vi "Two Parameter Marco Reparam EB only.vi"() -> ()   [LabVIEW 2015]
uses:
  <vilib>/Platform/TimedLoop/XDataNode/timing_clust.ctl
  <vilib>/Platform/TimedLoop/XDataNode/nitl_modes.ctl
  <vilib>/Platform/TimedLoop/XDataNode/wakeup.ctl
  <vilib>/DAQmx/read.llb/DAQmx Read (Analog DBL 1Chan 1Samp).vi
  <vilib>/DAQmx/read.llb/DAQmx Read (Analog 1D DBL NChan 1Samp).vi
  <vilib>/DAQmx/create/channels.llb/DAQmx Create Channel (AI-Voltage-Basic).vi
  <vilib>/Enthought/Python Integration Toolkit/api/Unpack Double.vi
  <vilib>/DAQmx/miscellaneous.llb/DAQmx Fill In Error Info.vi
  <vilib>/Platform/TimedLoop/XDataNode/XDataNode.xnode
  Program Files/neMESYS_SDK/neMESYS LabVIEW Kit/neMESYS LabVIEW Integration Kit.lvlib
  <vilib>/Platform/TimedLoop/XDataNode/XDNodeRunTimeDep.lvlib
  Conor/Temp CN7500/Omega CN7500/Omega CN7500.lvlib
  <vilib>/Enthought/Python Integration Toolkit/Python Integration Toolkit.lvlib
panel:
  out "Exp 10":bool
  out "Temp 3":dbl
  out "Flow 3":dbl
  out "Conc 3":dbl
  out "C BAcid 2":dbl
  out "C EB 2":dbl
  in  "Temp 3":dbl
  in  "Conc 3":dbl
  in  "Flow 3":dbl
  in  "LogFileName must end with .txt":string
  out "Param 1 8":dbl
  out "T value 1 8":dbl
  out "Param 2 8":dbl
  out "T value 2 8":dbl
  out "T Ref 8":dbl
  out "Correlation 8":dbl
  out "X2 8":dbl
  out "X2 ref 8":dbl
  out "Temp 9":dbl
  out "Flow 9":dbl
  out "Conc 9":dbl
  out "C BAcid 8":dbl
  out "C EB 8":dbl
  out "Exp 9":bool
  out "Param 1 7":dbl
  out "T value 1 7":dbl
  out "Param 2 7":dbl
  out "T value 2 7":dbl
  out "T Ref 7":dbl
  out "Correlation 7":dbl
  out "X2 7":dbl
  out "X2 ref 7":dbl
  out "Temp 8":dbl
  out "Flow 8":dbl
  out "Conc 8":dbl
  out "C BAcid 7":dbl
  out "C EB 7":dbl
  out "Exp 8":bool
  out "Param 1 6":dbl
  out "T value 1 6":dbl
  out "Param 2 6":dbl
  out "T value 2 6":dbl
  out "T Ref 6":dbl
  out "Correlation 6":dbl
  out "X2 6":dbl
  out "X2 ref 6":dbl
  out "Temp 7":dbl
  out "Flow 7":dbl
  out "Conc 7":dbl
  out "C BAcid 6":dbl
  out "C EB 6":dbl
  out "Exp 7":bool
  out "Param 1 5":dbl
  out "T value 1 5":dbl
  out "Param 2 5":dbl
  out "T value 2 5":dbl
  out "T Ref 5":dbl
  out "Correlation 5":dbl
  out "X2 5":dbl
  out "X2 ref 5":dbl
  out "Temp 6":dbl
  out "Flow 6":dbl
  out "Conc 6":dbl
  out "C BAcid 5":dbl
  out "C EB 5":dbl
  out "Exp 6":bool
  out "Param 1 4":dbl
  out "T value 1 4":dbl
  out "Param 2 4":dbl
  out "T value 2 4":dbl
  out "T Ref 4":dbl
  out "Correlation 4":dbl
  out "X2 4":dbl
  out "X2 ref 4":dbl
  out "Temp 5":dbl
  out "Flow 5":dbl
  out "Conc 5":dbl
  out "C BAcid 4":dbl
  out "C EB 4":dbl
  out "Exp 5":bool
  out "Param 1 3":dbl
  out "T value 1 3":dbl
  out "Param 2 3":dbl
  out "T value 2 3":dbl
  out "T Ref 3":dbl
  out "Correlation 3":dbl
  out "X2 3":dbl
  out "X2 ref 3":dbl
  out "Temp 4":dbl
  out "Flow 4":dbl
  out "Conc 4":dbl
  out "C BAcid 3":dbl
  out "C EB 3":dbl
  out "Exp 4":bool
  out "Conc 10":dbl
  out "Flow 10":dbl
  out "Temp 10":dbl
  in  "Design Criteria A or D or E or SV":string
  in  "Reparameterise? ON or OFF":string
  out "Exp 2":bool
  out "C EB 1":dbl
  out "C BAcid 1":dbl
  out "X2 ref 9":dbl
  out "X2 9":dbl
  out "Exp 2":bool
  out "Liquid Inlet Pressure (bar g)":dbl
  in  "Liquid P sensor Terminal Configuration":i32(ring)=-1 items=["default"=-1, "RSE"=10083, "NRSE"=10078, "Differential"=10106, "Pseudodifferential"=12529]
  in  "Liquid P sensor Physical Channel":tag="Dev1/ai0"
  in  "Temp 2":dbl
  in  "Conc 2":dbl
  in  "Flow 2":dbl
  out "Correlation 9":dbl
  out "T Ref 9":dbl
  out "Exp Finish":bool
  out "Exp 1":bool
  out "Exp 0":bool
  out "Conc 1":dbl
  out "Flow 1":dbl
  out "Temp 1":dbl
  out "Conc 2":dbl
  out "Flow 2":dbl
  out "Temp 2":dbl
  out "Param 1 9":dbl
  out "T value 1 9":dbl
  out "Param 2 9":dbl
  out "T value 2 9":dbl
  out "C BAcid 9":dbl
  out "C EB 9":dbl
  in  "Result file name must end with .xlsx":string
  in  "HPLC file Name, dont need extension":string
  out "Desired Conc Not Possible":bool
  in  "Safety or Emergency Syringe Control":bool
  out "Feed Concentration (M)":dbl
  out "Total Flowrate (uL/min)":dbl
  out "Gas Back Pressure (barg)":dbl
  in  "Shut down in empty?\nLeft off, right on":bool
  in  "Clear":bool
  out "Safety Shut Down Pressure (barg)":dbl
  out "Calculated Pressure":dbl[](graph)
  out "Safety Shut Down Temp":dbl
  out "Actual Temp (oC)":dbl
  out "Temperature":dynamicdata(graph)
  out "Temp Set Point (oC)":dbl
  in  "Temp 1":dbl
  in  "Temp 0":dbl
  in  "Update Temperature Set Point":bool
  in  "Automated Experiments or Direct Control":bool
  in  "Set Point (oC)":dbl
  out "loop ind":dbl
  in  "Stop everything":bool
  in  "Skip Exp":bool
  in  "Minutes between Exp":dbl min=0.0 step=0.05
  in  "Refill 4":bool
  in  "Refill 3":bool
  in  "Refill 2":bool
  in  "Refill 1":bool
  in  "Empty 4":bool
  in  "Empty 3":bool
  in  "Empty 2":bool
  in  "Empty 1":bool
  in  "Calibrate 4":bool
  in  "Calibrate 3":bool
  in  "Calibrate 2":bool
  in  "Calibrate 1":bool
  in  "Stop Dose 4":bool
  in  "Stop Dose 3":bool
  in  "Stop Dose 2":bool
  in  "Stop Dose 1":bool
  in  "Flow 1":dbl
  in  "Conc 1":dbl
  in  "Flow 0":dbl
  in  "Conc 0":dbl
  in  "Generate Flow":bool
  in  "Set Flowrate 1":dbl
  in  "Set Flowrate 2":dbl
  in  "Set Flowrate 3":dbl
  in  "Set Flowrate 4":dbl
  in  "High Conc":dbl min=0.0 max=2.0
  in  "Low Conc":dbl min=0.0 max=2.0
  out "Volumetric Fraction Acid":dbl min=0.0 max=1.0
  out "Syringe Level 4":dbl(slide) scale=0.0..5500.0
  out "Syringe Level 3":dbl(slide) scale=0.0..5500.0
  out "Syringe Level 2":dbl(slide) scale=0.0..5500.0
  out "Syringe Level 1":dbl(slide) scale=0.0..5500.0
  out "Flowrate 4 Ethanol":dbl
  out "Flowrate 3 Acid":dbl
  out "Flowrate 2 High":dbl
  out "Flowrate 1 Low":dbl
  # "Pre Planned Experiments"
  # "Conducted Experiments Set Points"
  # "Safety (start and end)"
  # "Current Conditions"
  # "(uL/min)"
  # "Coerced to nearest possible"
  # "Experimental Info"
  # "Acid must be between 0 and 1, normally 0.1 for 10%"
  # "Direct Control"
  # "Unit of Gas Flow NmL/min"
  # "I swapped syringe 1 and 2, so now 2 is high and 1 is low"
  # "Emergency Syringe Control Below"
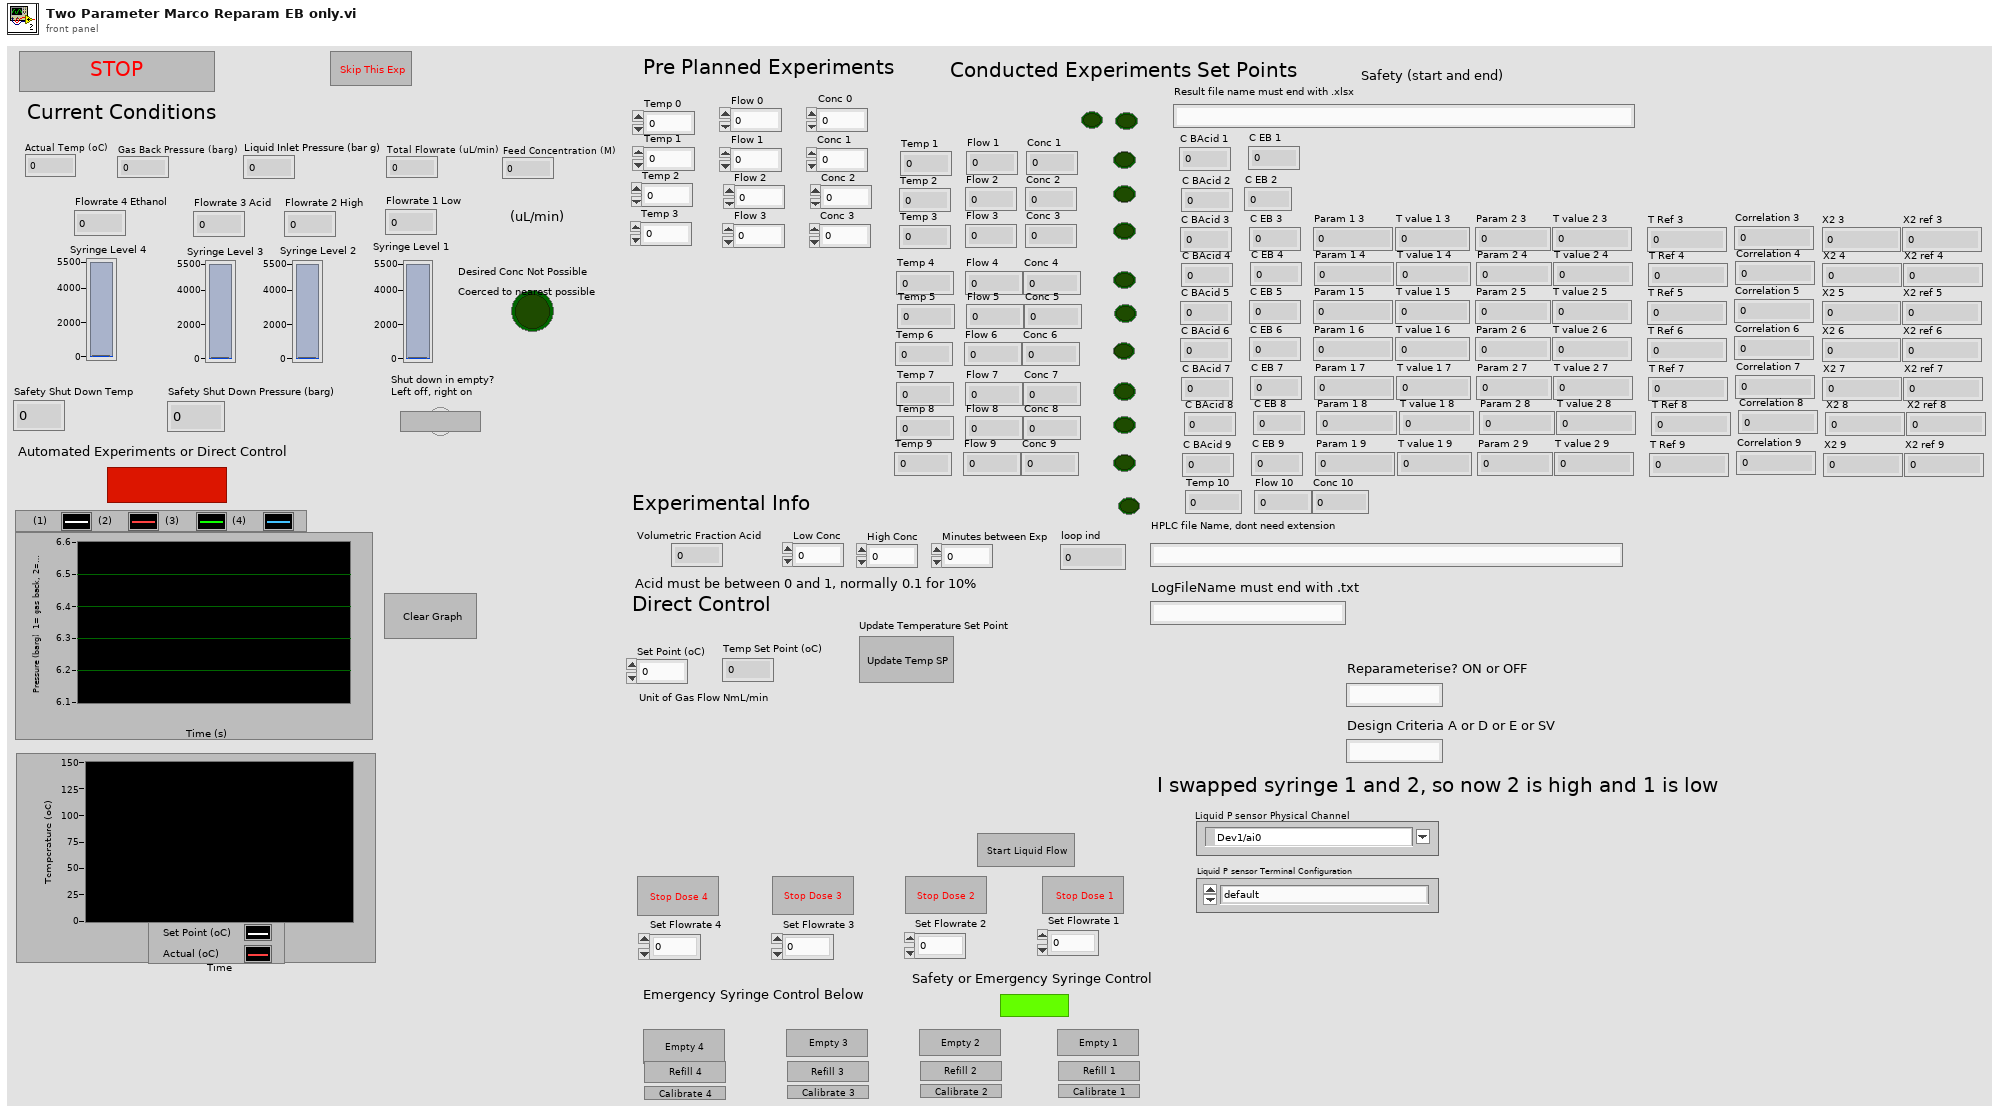
[diagram p1: front panel]
types:
  T1 = typedef "XDNodeRunTimeDep.lvlib/timing_clust.ctl" = cluster{"Expected End [f-1]":u64, "Actual End [f-1]":u64, "Finished Late? [f-1]":bool, "Expected End [i-1]":u64, "Actual End [i-1]":u64, "Finished Late? [i-1]":bool, "Expected Start [i]":u64, "Actual Start [i]":u64, "Expected Start [f]":u64, "Actual Start [f]":u64, "Source Name":string, "Structure Name":string, "Period":i64, "Deadline":i64, "Offset":i64, "Start":i64, "Priority":i32, "Timeout":i32, "Mode":T2, "Wakeup Reason":T3, "Error":errorcluster, "Source Type":string, "Secondary Source Type":string, "Global End Time":u64, "Global Start Time":u64, "Frame Duration":u64, "Iteration Duration":u64, "Assigned CPU":i32, "I/O Scan Engine Mode":u32}
  T2 = typedef "XDNodeRunTimeDep.lvlib/nitl_modes.ctl" = enum32{"No Change", "Process missed periods, maintain original phase", "Discard missed periods, maintain original phase", "Process missed periods, ignore original phase", "Discard missed periods, ignore original phase"}
  T3 = typedef "XDNodeRunTimeDep.lvlib/wakeup.ctl" = enum32{"Normal", "Aborted", "Asynchronous wakeup", "Timing source error", "Timed loop error", "Timeout"}
  T4 = typedef "Python Integration Toolkit.lvlib/Session ID.ctl" = u64
  T5 = typedef "Python Integration Toolkit.lvlib/Python Objects.ctl" = variant
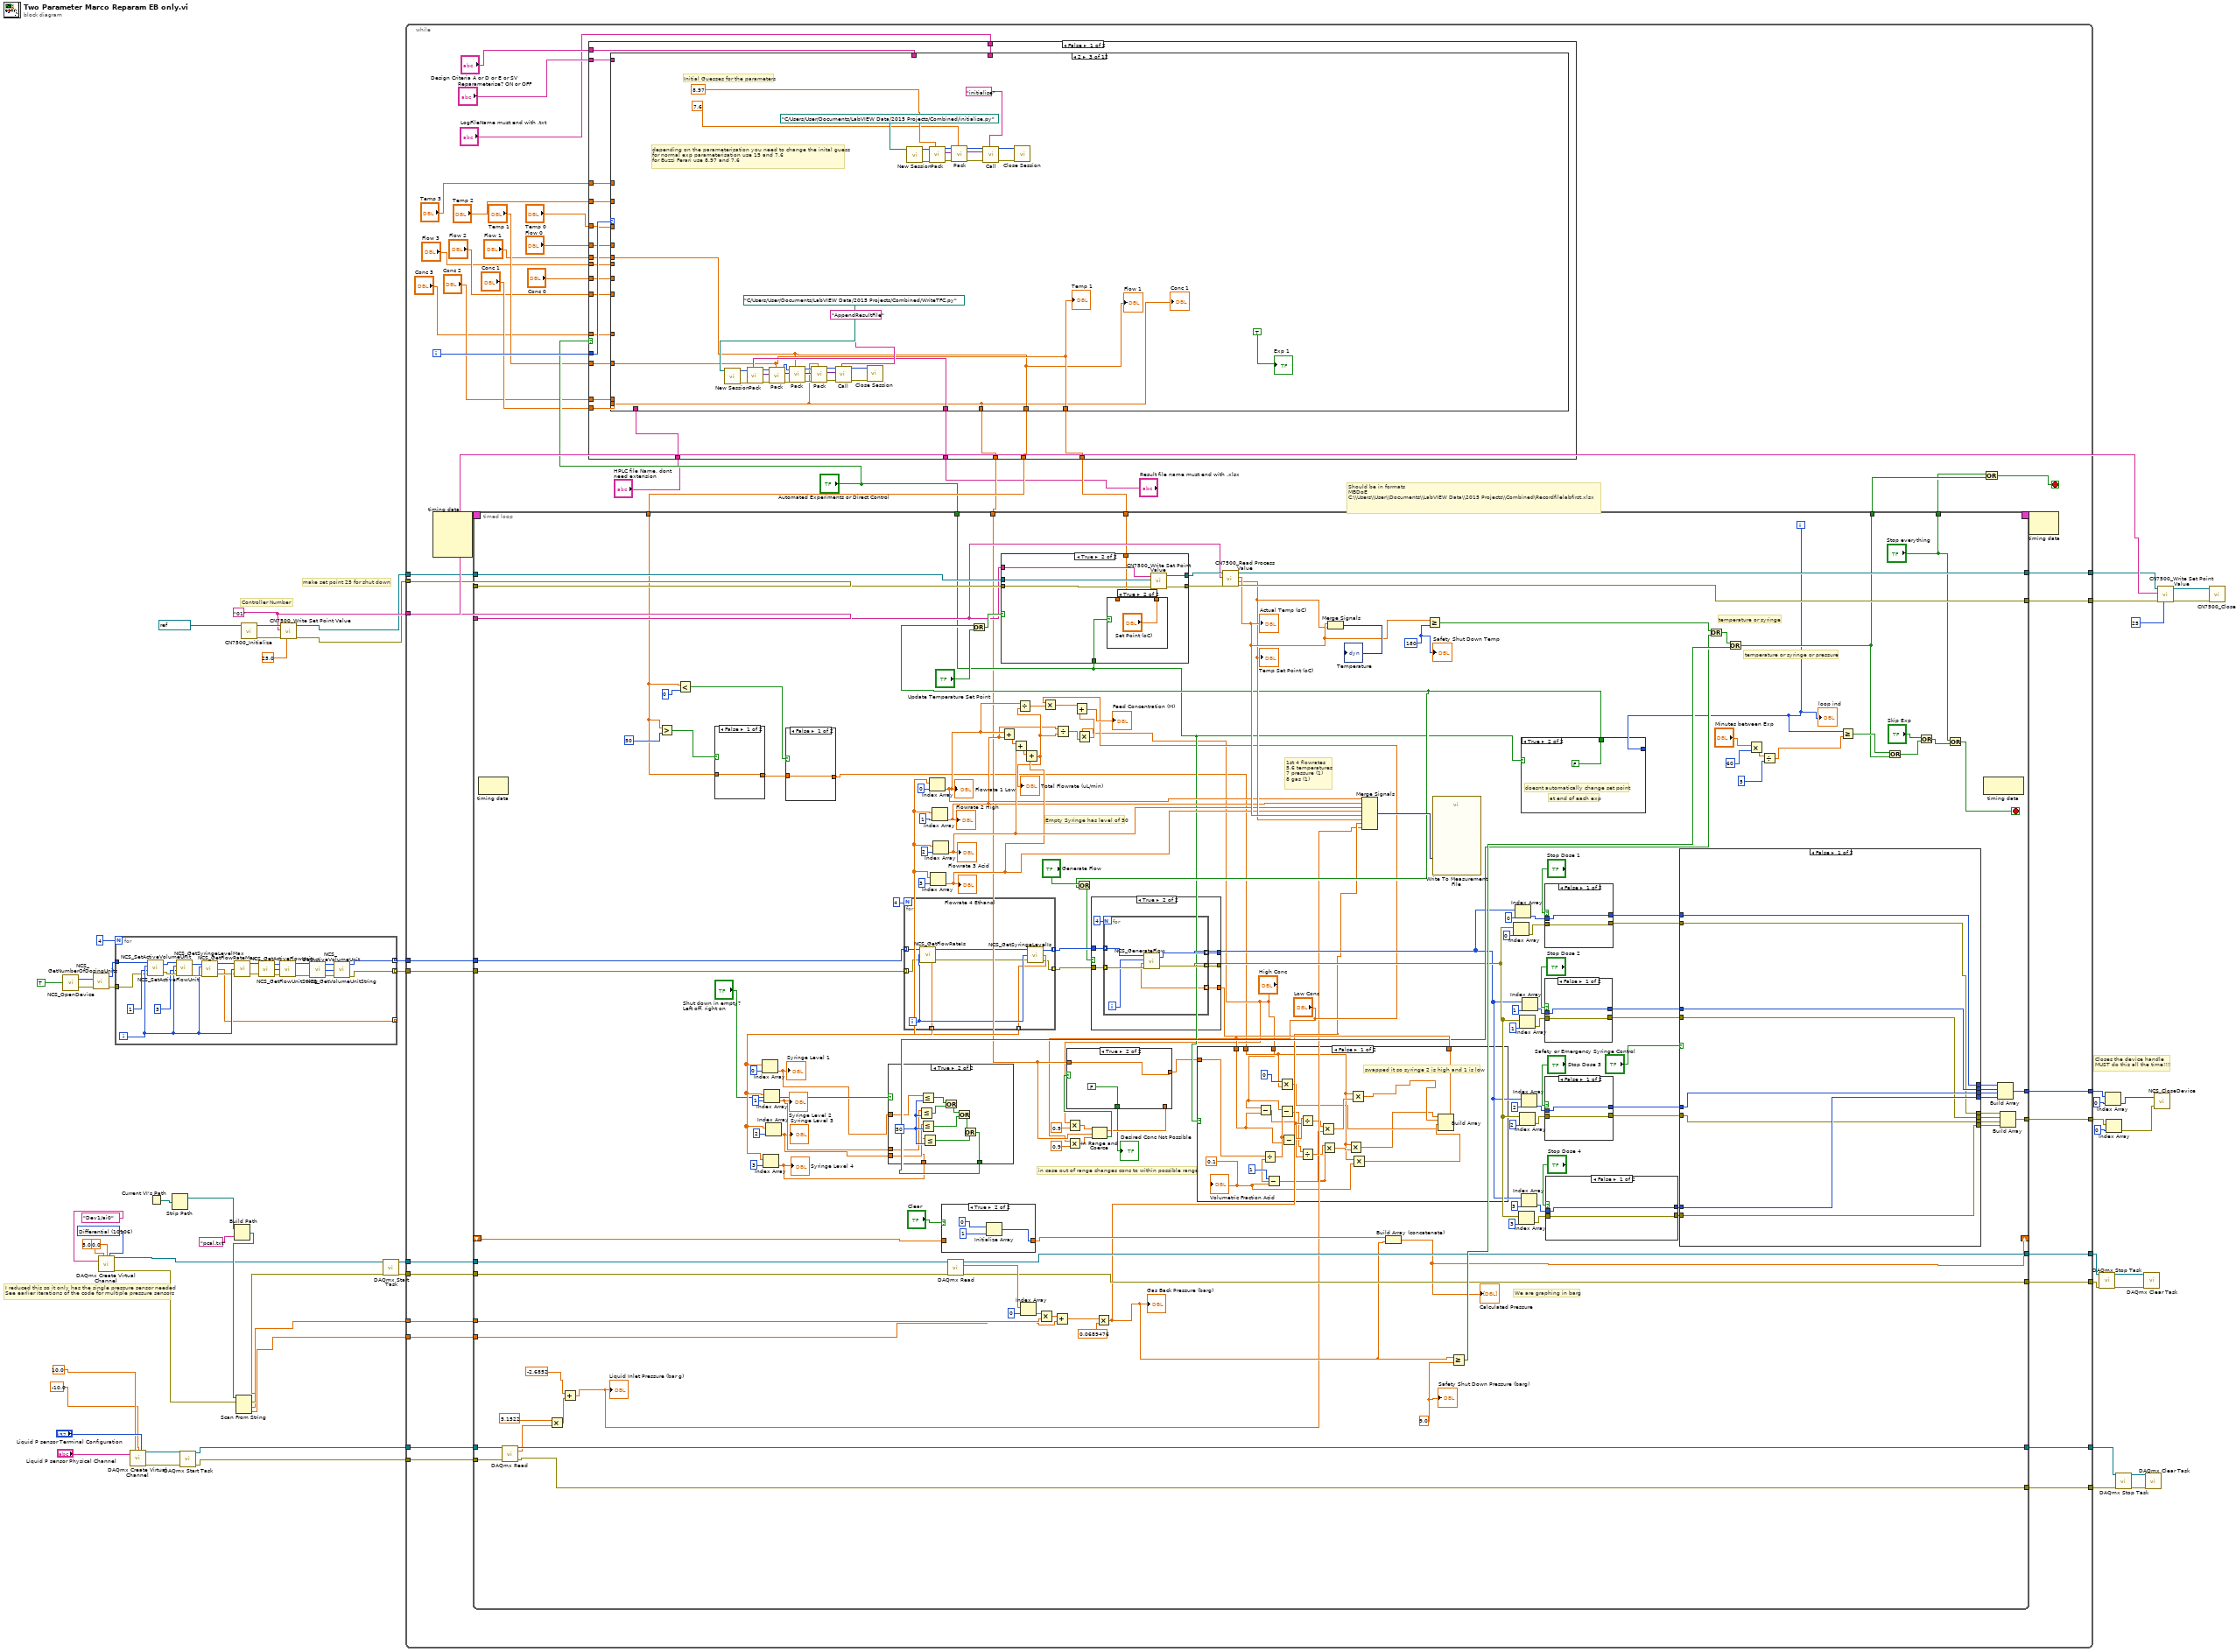
[diagram p0: block diagram]
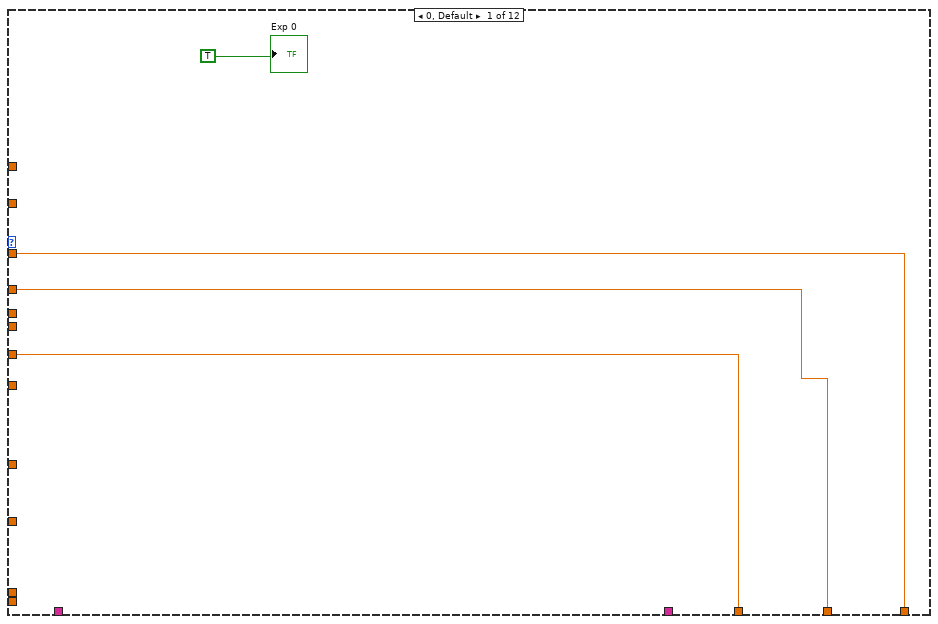
[diagram p2: hidden frame]
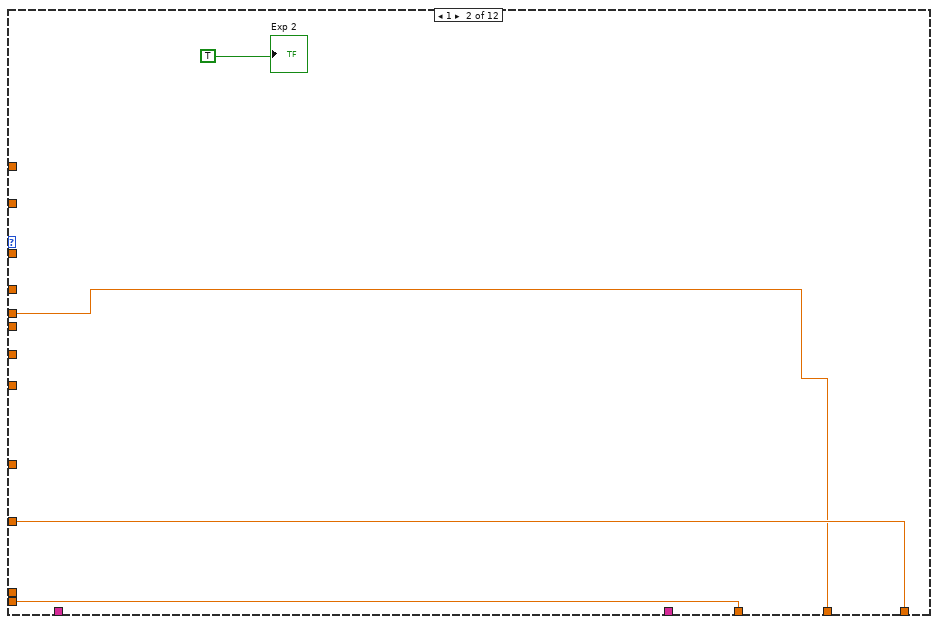
[diagram p3: hidden frame]
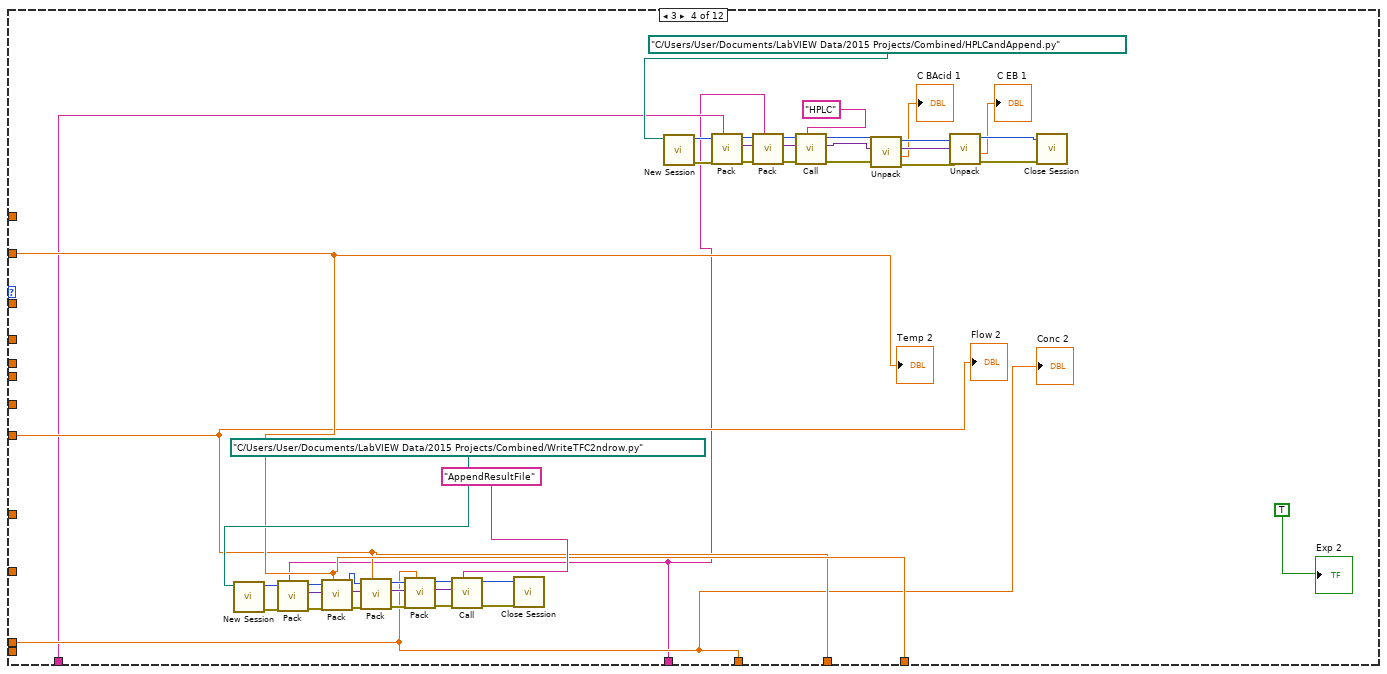
[diagram p4: hidden frame]
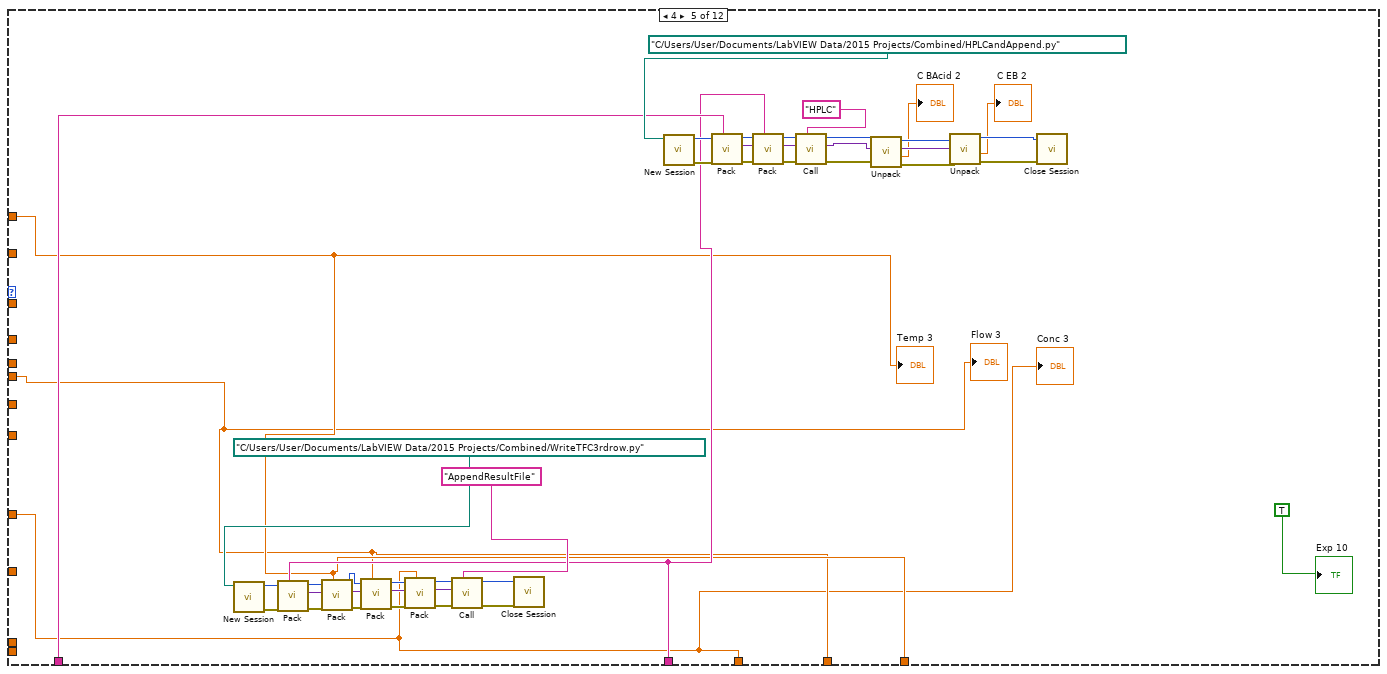
[diagram p5: hidden frame]
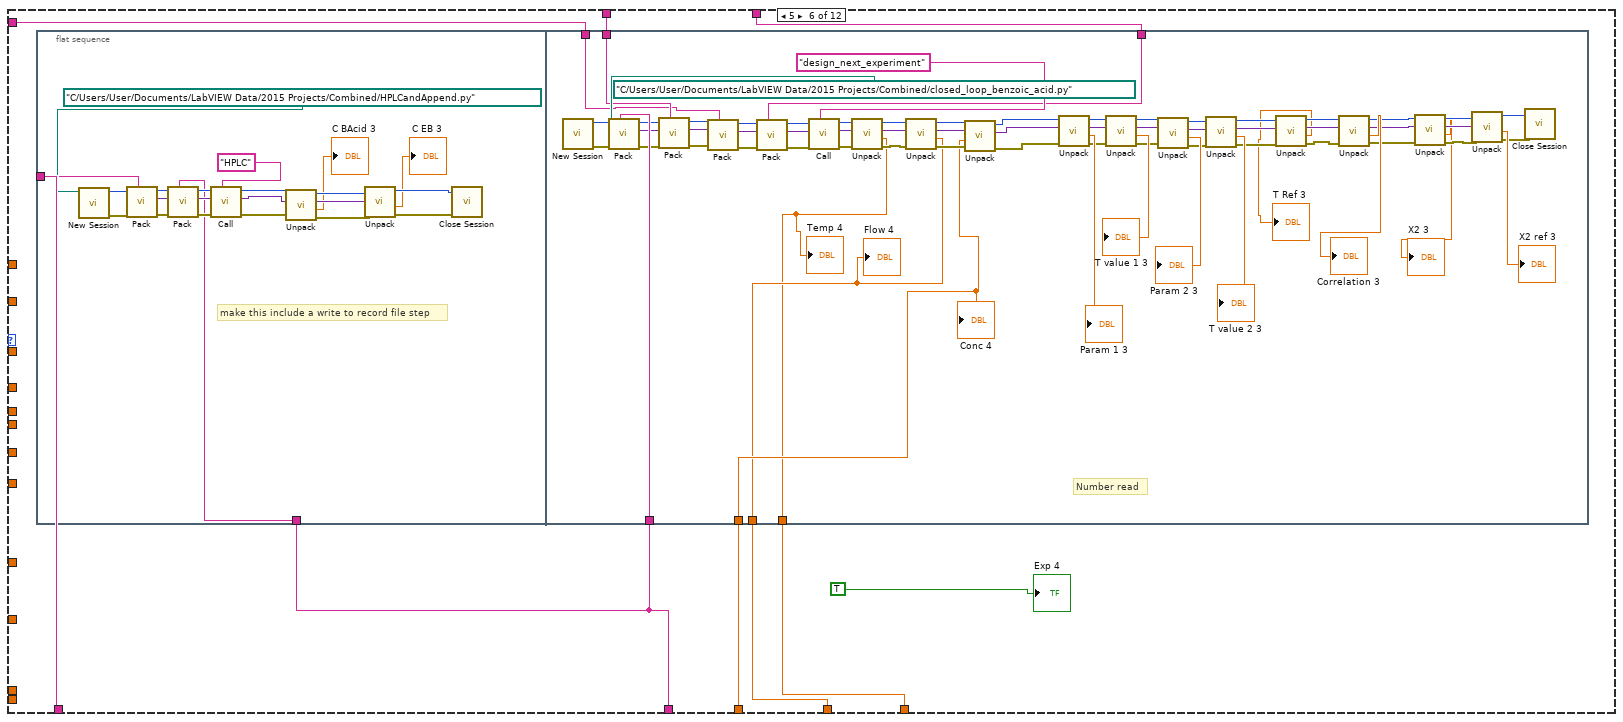
[diagram p6: hidden frame]
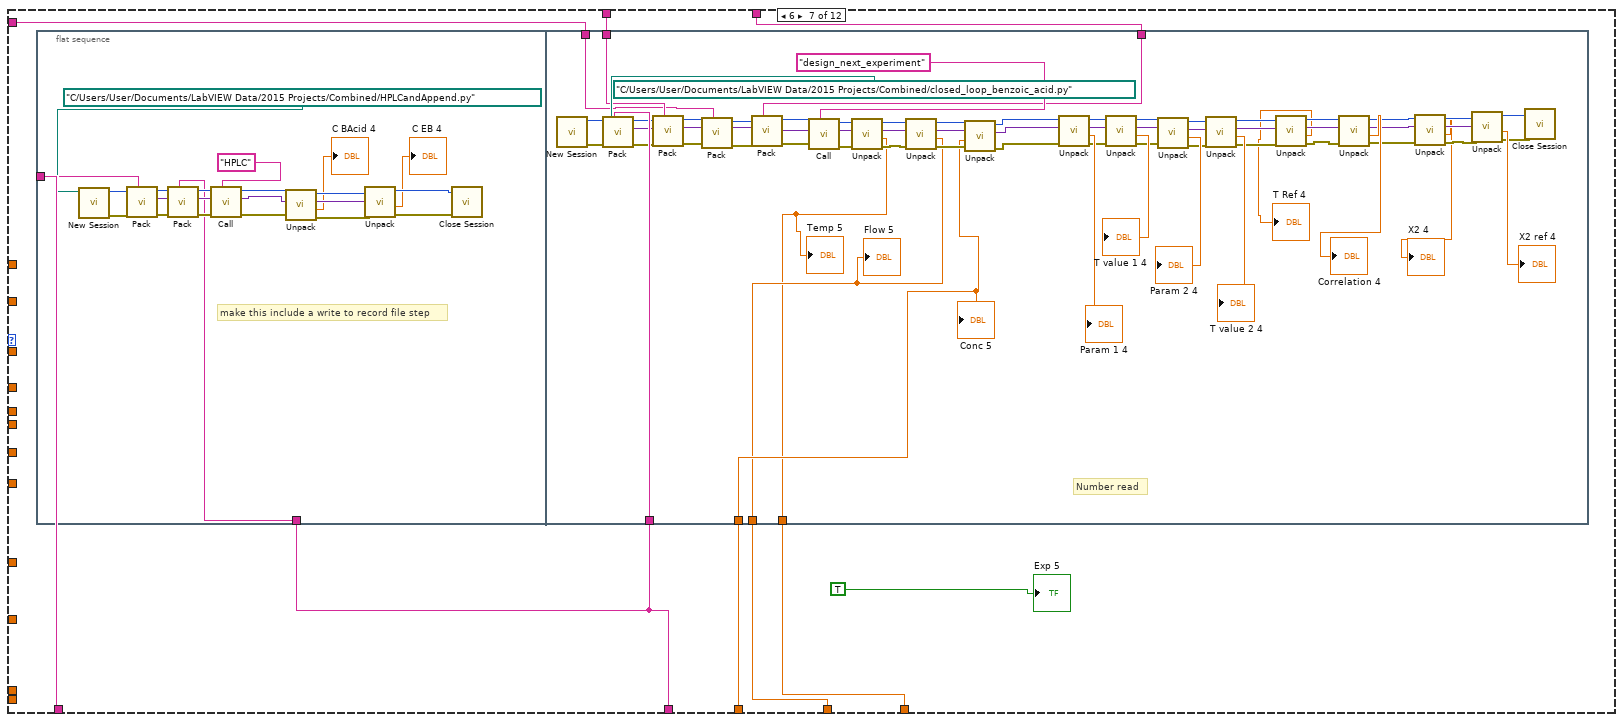
[diagram p7: hidden frame]
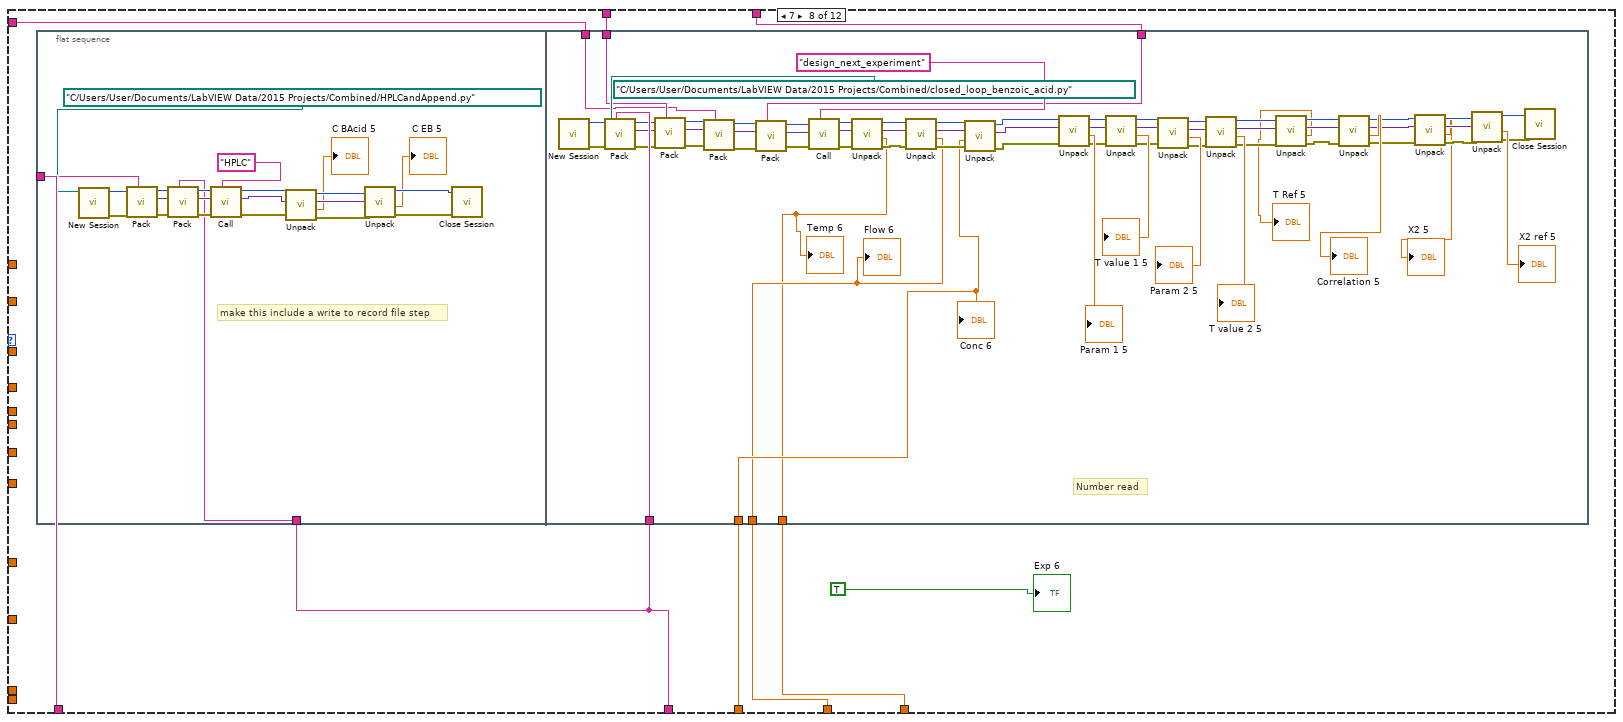
[diagram p8: hidden frame]
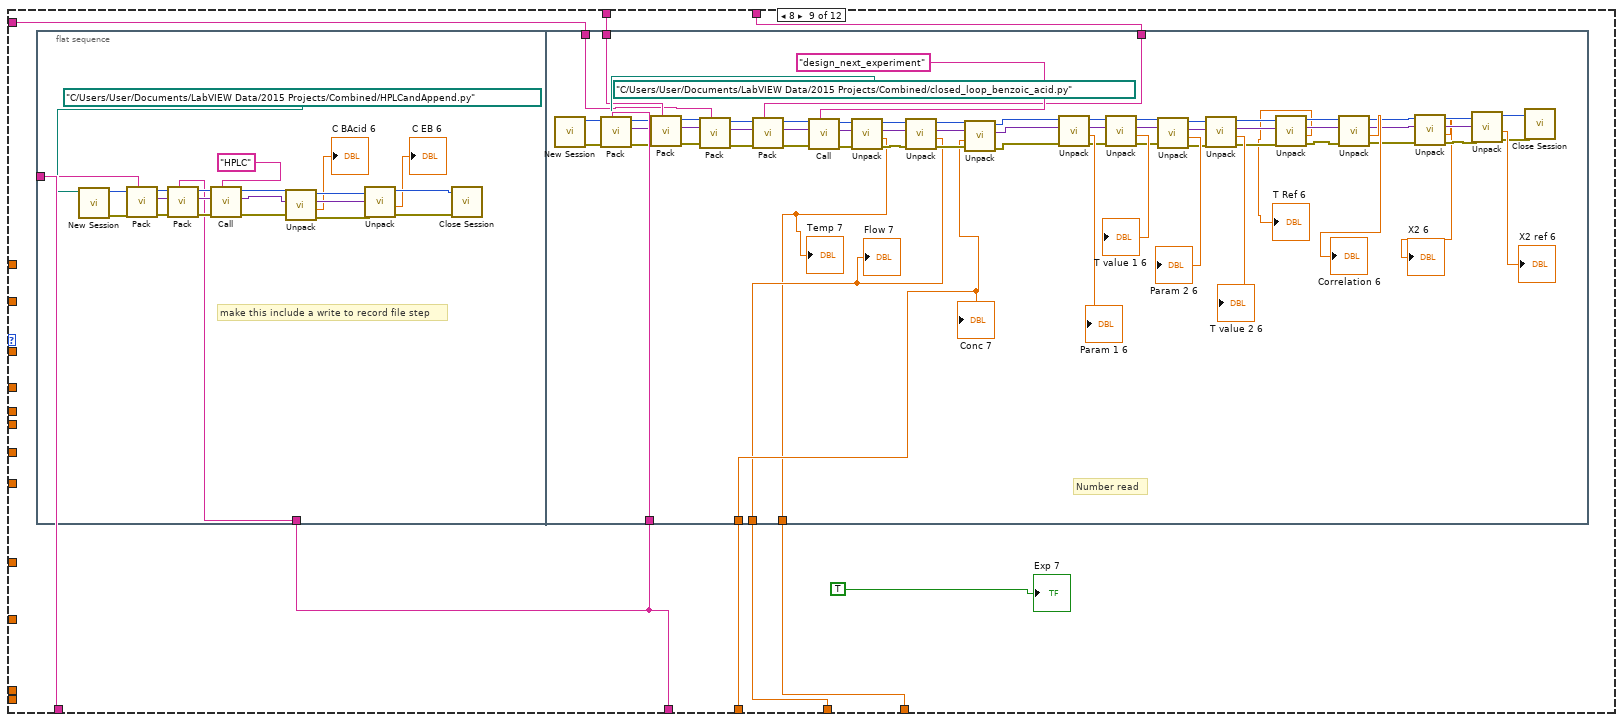
[diagram p9: hidden frame]
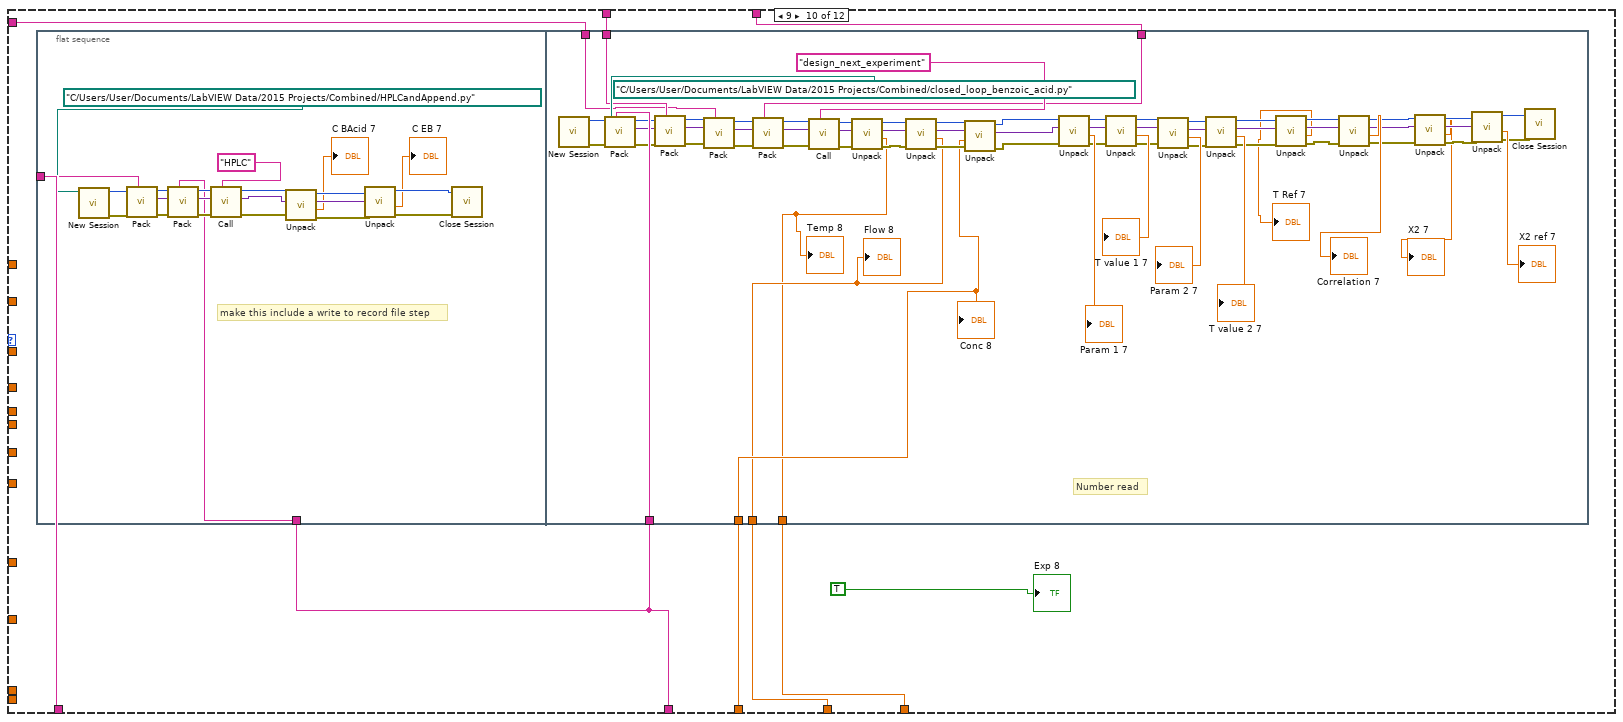
[diagram p10: hidden frame]
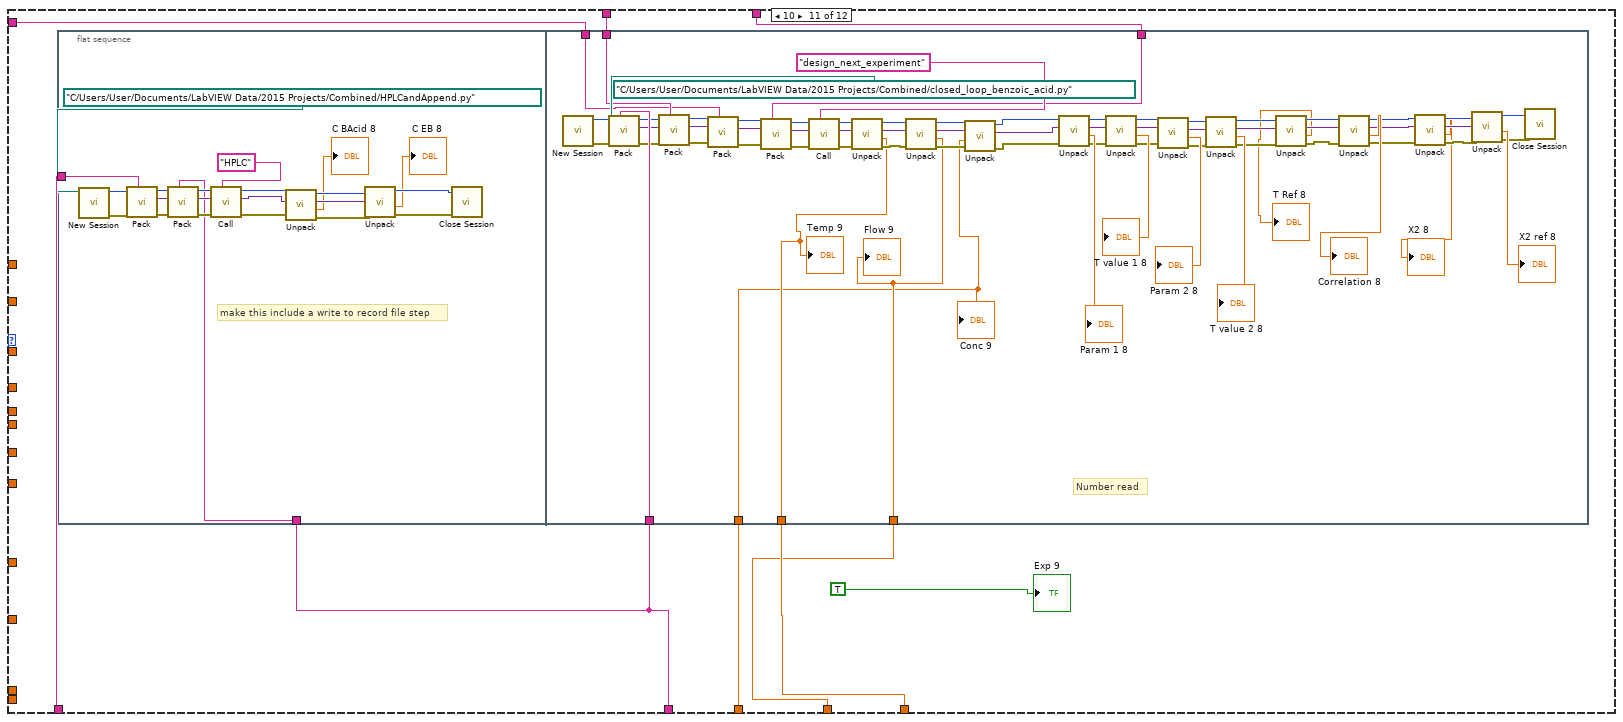
[diagram p11: hidden frame]
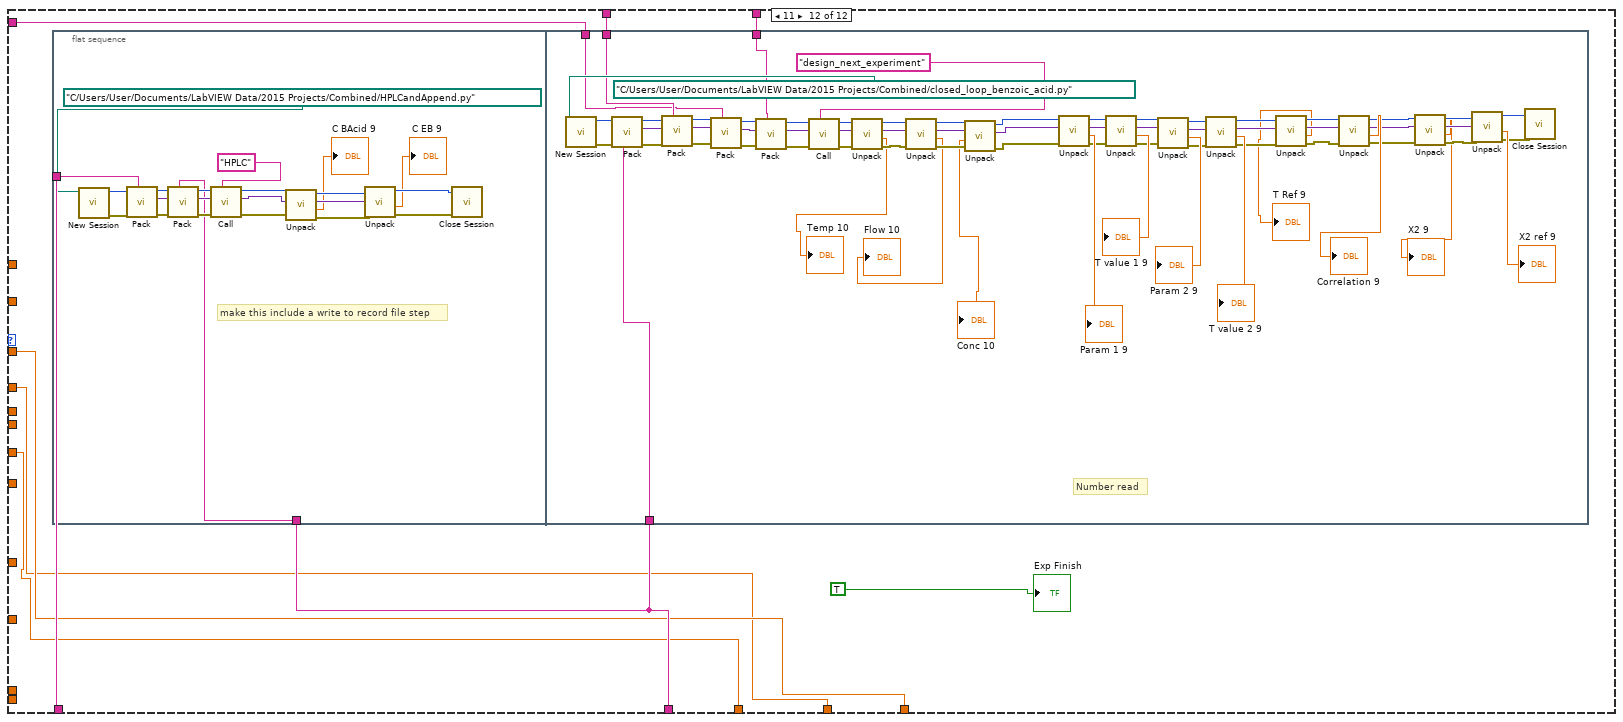
[diagram p12: hidden frame]
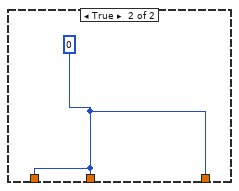
[diagram p13: hidden frame]
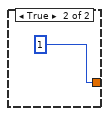
[diagram p14: hidden frame]
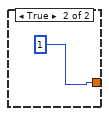
[diagram p15: hidden frame]
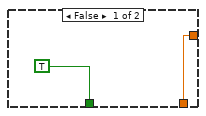
[diagram p16: hidden frame]
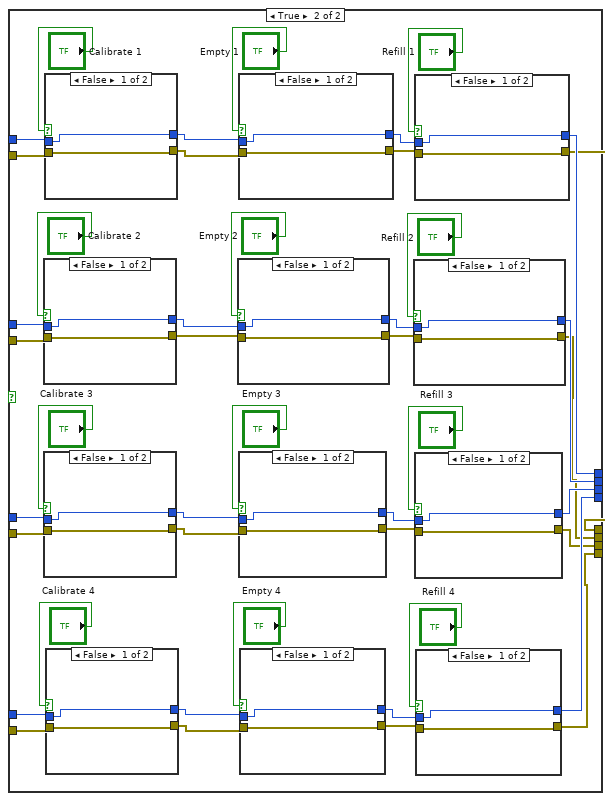
[diagram p17: hidden frame]
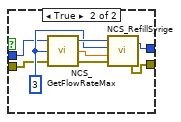
[diagram p18: hidden frame]
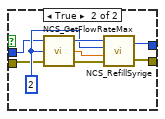
[diagram p19: hidden frame]
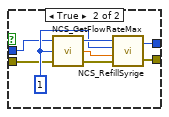
[diagram p20: hidden frame]
diagram:
  w29 = 10106 items=["default"=-1, "RSE"=10083, "NRSE"=10078, "Differential"=10106, "Pseudodifferential"=12529] ("input terminal configuration")
  w36 = "01" ("Controller Number")
  # "I reduced this so it only has the single pressure sensor needed\nSee earlier iterations of the code for multiple pressure sensors"
  # "make set point 25 for shut down"
  # "Controller Number"
  # "Closes the device handle \nMUST do this all the time!!!!"
  n1 = call "NCS_OpenDevice.vi"("show status window"=TRUE) -> ("device handle"=w55:u32, "error out"=w54:errorcluster)
  n2 = call "NCS_GetNumberOfDosingUnits.vi"("device handle in"=w55, "error in (no error)"=w54) -> ("device handle out"=w52:u32, "error out"=w53:errorcluster)  [unwired: 1 out]
  n3 = call-poly <vilib>:"DAQmx Create Virtual Channel.vi"("maximum value"=5.0, "minimum value"=0.0, "input terminal configuration"=w29, "physical channels"=tag "Dev1/ai0") -> ("task out"=w13:refnum<k21>, "error out"=w14:errorcluster)  [unwired: 10 in]
  n4 = for {
    N: 4 -> [_]
    tunnel: [w61] -> w51 mode=indexing
    tunnel: [w60] -> w50 mode=indexing
    tunnel: [w74] -> _ mode=indexing
    tunnel: w53 -> [w59]
    tunnel: w52 -> [w58]
    i -> [w77]
    n5 = call "NCS_SetActiveVolumeUnit.vi"("error in (no error)"=w59, "active volume unit"=1, "dosingunit"=w77, "device handle in"=w58) -> ("error out"=w80:errorcluster, "device handle out"=w81:u32)
    n6 = call "NCS_SetActiveFlowUnit.vi"("error in (no error)"=w80, "active flow unit"=3, "dosingunit"=w77, "device handle in"=w81) -> ("error out"=w78:errorcluster, "device handle out"=w79:u32)
    n7 = call "NCS_GetSyringeLevelMax.vi"("error in (no error)"=w78, "dosingunit"=w77, "device handle in"=w79) -> ("error out"=w75:errorcluster, "syringe level max"=w74:dbl, "device handle out"=w76:u32)  [unwired: 1 out]
    n8 = call "NCS_GetFlowRateMax.vi"("error in (no error)"=w75, "dosingunit"=w77, "device handle in"=w76) -> ("error out"=w62:errorcluster, "device handle out"=w63:u32)  [unwired: 1 out]
    n9 = call "NCS_GetActiveFlowUnit.vi"("error in (no error)"=w62, "device handle in"=w63) -> ("error out"=w70:errorcluster, "active flow unit"=w69:u8, "device handle out"=w71:u32)  [unwired: 1 in]
    n10 = call "NCS_GetFlowUnitString.vi"("device handle in"=w71, "flow unit id"=w69, "error in (no error)"=w70) -> ("device handle out"=w66:u32, "error out"=w65:errorcluster)  [unwired: 2 out]
    n11 = call "NCS_GetActiveVolumeUnit.vi"("error in (no error)"=w65, "device handle in"=w66) -> ("error out"=w67:errorcluster, "active volume unit"=w68:u8, "device handle out"=w64:u32)  [unwired: 1 in]
    n12 = call "NCS_GetVolumeUnitString.vi"("device handle in"=w64, "volume unit id"=w68, "error in (no error)"=w67) -> ("device handle out"=w61:u32, "error out"=w60:errorcluster)  [unwired: 2 out]
  }
  n13 = call-poly <vilib>:"DAQmx Create Virtual Channel.vi"("maximum value"=10.0, "minimum value"=-10.0 ("maximum value"), "input terminal configuration"="Liquid P sensor Terminal Configuration", "physical channels"="Liquid P sensor Physical Channel") -> ("task out"=w9:refnum<k21>, "error out"=w10:errorcluster)  [unwired: 10 in]
  n14 = Current VI's Path() -> (path=w27:path)
  n15 = Strip Path(path=w27) -> (stripped path=w25:path)  [unwired: 1 out]
  n16 = call <vilib>:"DAQmx Start Task.vi"("task/channels in"=w9, "error in"=w10) -> ("task out"=w8:refnum<k21>, "error out"=w7:errorcluster)  [unwired: 12 in]
  n17 = Build Path(base path=w25, name or relative path="pcal.txt") -> (appended path=w26:path)
  n18 = Scan From String(w26, w14) -> (w23:errorcluster, output 1=w20:dbl, output 2=w19:dbl)  [unwired: 3 in, 1 out]
  n19 = call "CN7500_Initialize.vi"("VISA resource name"=refnum<visa-resource-name> "COM8") -> ("error out"=w42:errorcluster, "VISA resource name out"=w43:refnum<visa-resource-name>)  [unwired: 9 in]
  n20 = call "CN7500_Write Set Point Value.vi"("Target Set Point Value"=25.0, "error in (no error)"=w42, "Controller Number"=w36, "VISA In"=w43) -> ("error out"=w34:errorcluster, "VISA Out"=w35:refnum<visa-resource-name>)  [unwired: 6 in]
  n21 = call <vilib>:"DAQmx Start Task.vi"("task/channels in"=w13, "error in"=w23) -> ("task out"=w22:refnum<k21>, "error out"=w21:errorcluster)  [unwired: 12 in]
  n22 = while {
    tunnel: w51 -> [w127]
    tunnel: w50 -> [w126]
    tunnel: [w125] -> w45
    tunnel: [w124] -> w44
    tunnel: w36 -> [w121]
    tunnel: w35 -> [w120]
    tunnel: w34 -> [w119]
    tunnel: [w118] -> w33
    tunnel: [w117] -> w32
    tunnel: w22 -> [w115]
    tunnel: w21 -> [w114]
    tunnel: w20 -> [w113]
    tunnel: w19 -> [w112]
    tunnel: [w111] -> w16
    tunnel: [w110] -> w15
    tunnel: w8 -> [w94]
    tunnel: w7 -> [w93]
    tunnel: [w92] -> w5
    tunnel: [w91] -> w3
    i -> [w104]
    stop <- w109 stop-if-true
    # "Should be in formats \nMBDoE\nC:\\\\Users\\\\User\\\\Documents\\\\LabVIEW Data\\\\2015 Projects\\\\Combined\\Recordfilelabfirst.xlsx"
    n23 = node-c288() -> (w123:T1)  [unwired: 4 in]
    n24 = case shown="False" "Automated Experiments or Direct Control" {
      tunnel: [w145 w961] -> w107
      tunnel: [w143 w961] -> w106
      tunnel: [w147 w961] -> w105
      tunnel: w104 -> [w148 _]
      tunnel: "Conc 0" -> [w146 _]
      tunnel: "Flow 0" -> [w142 _]
      tunnel: "Temp 0" -> [w144 _]
      tunnel: "Temp 1" -> [w140 _]
      tunnel: "Flow 1" -> [w139 _]
      tunnel: "Conc 1" -> [w138 _]
      tunnel: "HPLC file Name, dont need extension" -> [w137 _]
      tunnel: "Result file name must end with .xlsx" -> [w141 _]
      tunnel: "Temp 2" -> [w136 _]
      tunnel: "Flow 2" -> [w135 _]
      tunnel: "Conc 2" -> [w134 _]
      tunnel: "Design Criteria A or D or E or SV" -> [w133 _]
      tunnel: "Reparameterise? ON or OFF" -> [w132 _]
      tunnel: "LogFileName must end with .txt" -> [w131 _]
      tunnel: "Temp 3" -> [w130 _]
      tunnel: "Flow 3" -> [w129 _]
      tunnel: "Conc 3" -> [w128 _]
      frame False {
        n25 = case shown="2" w148 {
          tunnel: [w150 w153 w172 w216 w238 w285 w382 w479 w576 w673 w767 w864] -> w147
          tunnel: w146 -> [w150 _ _ _ _ _ _ _ _ _ _ w864]
          tunnel: [w152 w155 w174 w218 w240 w283 w380 w477 w574 w671 w769 w866] -> w145
          tunnel: w144 -> [w152 _ _ _ _ _ _ _ _ _ _ w866]
          tunnel: [w151 w154 w173 w217 w239 w284 w381 w478 w575 w672 w768 w865] -> w143
          tunnel: w142 -> [w151 _ _ _ _ _ _ _ _ _ _ w865]
          tunnel: w141 -> [_ _ w175 w194 w241 w289 w386 w483 w580 w677 w774 w871]
          tunnel: w140 -> [_ w155 w174 _ _ _ _ _ _ _ _ _]
          tunnel: w139 -> [_ w154 w173 _ _ _ _ _ _ _ _ _]
          tunnel: w138 -> [_ w153 w172 _ _ _ _ _ _ _ _ _]
          tunnel: w137 -> [_ _ _ w195 w242 w290 w387 w484 w581 w678 w775 w872]
          tunnel: w136 -> [_ _ _ w218 _ _ _ _ _ _ _ _]
          tunnel: w135 -> [_ _ _ w217 _ _ _ _ _ _ _ _]
          tunnel: w134 -> [_ _ _ w216 _ _ _ _ _ _ _ _]
          tunnel: w133 -> [_ _ _ _ _ w287 w384 w481 w578 w675 w772 w869]
          tunnel: w132 -> [_ _ _ _ _ w286 w383 w480 w577 w674 w771 w868]
          tunnel: w131 -> [_ _ _ _ _ w282 w379 w476 w573 w670 w770 w867]
          tunnel: w130 -> [_ _ _ _ w240 _ _ _ _ _ _ _]
          tunnel: w129 -> [_ _ _ _ w239 _ _ _ _ _ _ _]
          tunnel: w128 -> [_ _ _ _ w238 _ _ _ _ _ _ _]
          frame 0, Default {
            "Exp 0" <- TRUE
          }
          frame 1 {
            "Exp 2" <- TRUE
          }
          frame 2 {
            # "depending on the parameterisation you need to change the inital guess\nfor normal exp parameterisation use 15 and 7.6\nfor Buzzi Ferari use 8.97 and 7.6"
            # "Initial Guesses for the parameters"
            n26 = call <vilib>:"New Session.vi"("Path to Python Module (.py File)"=path "C:/Users/User/Documents/LabVIEW Data/2015 Projects/Combined/WriteTFC.py") -> ("error out"=w185:errorcluster, "Session ID out"=w184:T4)  [unwired: 9 in]
            n27 = call <vilib>:"Pack.vi"("Argument"=w175, "error in (no error)"=w185, "Session ID"=w184) -> ("error out"=w186:errorcluster, "Python Object References Out"=w190:T5, "Session ID out"=w183:T4)  [unwired: 6 in]
            n28 = call <vilib>:"Pack.vi"("Argument"=w174, "error in (no error)"=w186, "Python Object References In"=w190, "Session ID"=w183) -> ("error out"=w187:errorcluster, "Python Object References Out"=w191:T5, "Session ID out"=w193:T4)  [unwired: 5 in]
            n29 = call <vilib>:"Pack.vi"("Argument"=w173, "error in (no error)"=w187, "Python Object References In"=w191, "Session ID"=w193) -> ("error out"=w188:errorcluster, "Python Object References Out"=w192:T5, "Session ID out"=w179:T4)  [unwired: 5 in]
            n30 = call <vilib>:"Pack.vi"("Argument"=w172, "error in (no error)"=w188, "Python Object References In"=w192, "Session ID"=w179) -> ("error out"=w176:errorcluster, "Python Object References Out"=w177:T5, "Session ID out"=w178:T4)  [unwired: 5 in]
            n31 = call <vilib>:"Call.vi"("Function or Method Name"="AppendResultFile", "error in (no error)"=w176, "Python Object References In"=w177, "Session ID"=w178) -> ("error out"=w189:errorcluster, "Session ID out"=w180:T4)  [unwired: 5 in, 1 out]
            n32 = call <vilib>:"Close Session.vi"("error in (no error)"=w189, "Session ID"=w180) -> ()  [unwired: 9 in, 1 out]
            n33 = call <vilib>:"New Session.vi"("Path to Python Module (.py File)"=path "C:/Users/User/Documents/LabVIEW Data/2015 Projects/Combined/initialise.py") -> ("error out"=w165:errorcluster, "Session ID out"=w169:T4)  [unwired: 9 in]
            n34 = call <vilib>:"Pack.vi"("Argument"=8.97, "error in (no error)"=w165, "Session ID"=w169) -> ("error out"=w164:errorcluster, "Python Object References Out"=w162:T5, "Session ID out"=w168:T4)  [unwired: 6 in]
            n35 = call <vilib>:"Pack.vi"("Argument"=7.6, "error in (no error)"=w164, "Python Object References In"=w162, "Session ID"=w168) -> ("error out"=w163:errorcluster, "Python Object References Out"=w161:T5, "Session ID out"=w167:T4)  [unwired: 5 in]
            n36 = call <vilib>:"Call.vi"("Function or Method Name"="initialise", "error in (no error)"=w163, "Python Object References In"=w161, "Session ID"=w167) -> ("error out"=w170:errorcluster, "Session ID out"=w166:T4)  [unwired: 5 in, 1 out]
            n37 = call <vilib>:"Close Session.vi"("error in (no error)"=w170, "Session ID"=w166) -> ()  [unwired: 9 in, 1 out]
            "Temp 1" <- w174
            "Flow 1" <- w173
            "Conc 1" <- w172
            "Exp 1" <- TRUE
          }
          frame 3 {
            n38 = call <vilib>:"New Session.vi"("Path to Python Module (.py File)"=path "C:/Users/User/Documents/LabVIEW Data/2015 Projects/Combined/WriteTFC2ndrow.py") -> ("error out"=w229:errorcluster, "Session ID out"=w228:T4)  [unwired: 9 in]
            n39 = call <vilib>:"Pack.vi"("Argument"=w194, "error in (no error)"=w229, "Session ID"=w228) -> ("error out"=w230:errorcluster, "Python Object References Out"=w234:T5, "Session ID out"=w227:T4)  [unwired: 6 in]
            n40 = call <vilib>:"Pack.vi"("Argument"=w218, "error in (no error)"=w230, "Python Object References In"=w234, "Session ID"=w227) -> ("error out"=w231:errorcluster, "Python Object References Out"=w235:T5, "Session ID out"=w237:T4)  [unwired: 5 in]
            n41 = call <vilib>:"Pack.vi"("Argument"=w217, "error in (no error)"=w231, "Python Object References In"=w235, "Session ID"=w237) -> ("error out"=w232:errorcluster, "Python Object References Out"=w236:T5, "Session ID out"=w223:T4)  [unwired: 5 in]
            n42 = call <vilib>:"Pack.vi"("Argument"=w216, "error in (no error)"=w232, "Python Object References In"=w236, "Session ID"=w223) -> ("error out"=w220:errorcluster, "Python Object References Out"=w221:T5, "Session ID out"=w222:T4)  [unwired: 5 in]
            n43 = call <vilib>:"Call.vi"("Function or Method Name"="AppendResultFile", "error in (no error)"=w220, "Python Object References In"=w221, "Session ID"=w222) -> ("error out"=w233:errorcluster, "Session ID out"=w224:T4)  [unwired: 5 in, 1 out]
            n44 = call <vilib>:"Close Session.vi"("error in (no error)"=w233, "Session ID"=w224) -> ()  [unwired: 9 in, 1 out]
            n45 = call <vilib>:"New Session.vi"("Path to Python Module (.py File)"=path "C:/Users/User/Documents/LabVIEW Data/2015 Projects/Combined/HPLCandAppend.py") -> ("error out"=w212:errorcluster, "Session ID out"=w211:T4)  [unwired: 9 in]
            n46 = call <vilib>:"Pack.vi"("Argument"=w195, "error in (no error)"=w212, "Session ID"=w211) -> ("error out"=w197:errorcluster, "Python Object References Out"=w199:T5, "Session ID out"=w201:T4)  [unwired: 6 in]
            n47 = call <vilib>:"Pack.vi"("Argument"=w194, "error in (no error)"=w197, "Python Object References In"=w199, "Session ID"=w201) -> ("error out"=w196:errorcluster, "Python Object References Out"=w198:T5, "Session ID out"=w200:T4)  [unwired: 5 in]
            n48 = call <vilib>:"Call.vi"("Function or Method Name"="HPLC", "error in (no error)"=w196, "Python Object References In"=w198, "Session ID"=w200) -> ("error out"=w213:errorcluster, "Python Object References Out"=w204:T5, "Session ID out"=w205:T4)  [unwired: 5 in]
            n49 = call-poly <vilib>:"Unpack.vi"("error in (no error)"=w213, "Python Object References In"=w204, "Session ID"=w205) -> ("error out"=w214:errorcluster, "Value"=→"C BAcid 1":dbl, "Python Object References Out"=w209:T5, "Session ID out"=w208:T4)  [unwired: 5 in]
            n50 = call-poly <vilib>:"Unpack.vi"("error in (no error)"=w214, "Python Object References In"=w209, "Session ID"=w208) -> ("error out"=w215:errorcluster, "Value"=→"C EB 1":dbl, "Session ID out"=w210:T4)  [unwired: 5 in, 1 out]
            n51 = call <vilib>:"Close Session.vi"("error in (no error)"=w215, "Session ID"=w210) -> ()  [unwired: 9 in, 1 out]
            "Exp 2" <- TRUE
            "Temp 2" <- w218
            "Flow 2" <- w217
            "Conc 2" <- w216
          }
          frame 4 {
            n52 = call <vilib>:"New Session.vi"("Path to Python Module (.py File)"=path "C:/Users/User/Documents/LabVIEW Data/2015 Projects/Combined/WriteTFC3rdrow.py") -> ("error out"=w273:errorcluster, "Session ID out"=w272:T4)  [unwired: 9 in]
            n53 = call <vilib>:"Pack.vi"("Argument"=w241, "error in (no error)"=w273, "Session ID"=w272) -> ("error out"=w274:errorcluster, "Python Object References Out"=w278:T5, "Session ID out"=w271:T4)  [unwired: 6 in]
            n54 = call <vilib>:"Pack.vi"("Argument"=w240, "error in (no error)"=w274, "Python Object References In"=w278, "Session ID"=w271) -> ("error out"=w275:errorcluster, "Python Object References Out"=w279:T5, "Session ID out"=w281:T4)  [unwired: 5 in]
            n55 = call <vilib>:"Pack.vi"("Argument"=w239, "error in (no error)"=w275, "Python Object References In"=w279, "Session ID"=w281) -> ("error out"=w276:errorcluster, "Python Object References Out"=w280:T5, "Session ID out"=w267:T4)  [unwired: 5 in]
            n56 = call <vilib>:"Pack.vi"("Argument"=w238, "error in (no error)"=w276, "Python Object References In"=w280, "Session ID"=w267) -> ("error out"=w264:errorcluster, "Python Object References Out"=w265:T5, "Session ID out"=w266:T4)  [unwired: 5 in]
            n57 = call <vilib>:"Call.vi"("Function or Method Name"="AppendResultFile", "error in (no error)"=w264, "Python Object References In"=w265, "Session ID"=w266) -> ("error out"=w277:errorcluster, "Session ID out"=w268:T4)  [unwired: 5 in, 1 out]
            n58 = call <vilib>:"Close Session.vi"("error in (no error)"=w277, "Session ID"=w268) -> ()  [unwired: 9 in, 1 out]
            n59 = call <vilib>:"New Session.vi"("Path to Python Module (.py File)"=path "C:/Users/User/Documents/LabVIEW Data/2015 Projects/Combined/HPLCandAppend.py") -> ("error out"=w259:errorcluster, "Session ID out"=w258:T4)  [unwired: 9 in]
            n60 = call <vilib>:"Pack.vi"("Argument"=w242, "error in (no error)"=w259, "Session ID"=w258) -> ("error out"=w244:errorcluster, "Python Object References Out"=w246:T5, "Session ID out"=w248:T4)  [unwired: 6 in]
            n61 = call <vilib>:"Pack.vi"("Argument"=w241, "error in (no error)"=w244, "Python Object References In"=w246, "Session ID"=w248) -> ("error out"=w243:errorcluster, "Python Object References Out"=w245:T5, "Session ID out"=w247:T4)  [unwired: 5 in]
            n62 = call <vilib>:"Call.vi"("Function or Method Name"="HPLC", "error in (no error)"=w243, "Python Object References In"=w245, "Session ID"=w247) -> ("error out"=w260:errorcluster, "Python Object References Out"=w251:T5, "Session ID out"=w252:T4)  [unwired: 5 in]
            n63 = call-poly <vilib>:"Unpack.vi"("error in (no error)"=w260, "Python Object References In"=w251, "Session ID"=w252) -> ("error out"=w261:errorcluster, "Value"=→"C BAcid 2":dbl, "Python Object References Out"=w256:T5, "Session ID out"=w255:T4)  [unwired: 5 in]
            n64 = call-poly <vilib>:"Unpack.vi"("error in (no error)"=w261, "Python Object References In"=w256, "Session ID"=w255) -> ("error out"=w262:errorcluster, "Value"=→"C EB 2":dbl, "Session ID out"=w257:T4)  [unwired: 5 in, 1 out]
            n65 = call <vilib>:"Close Session.vi"("error in (no error)"=w262, "Session ID"=w257) -> ()  [unwired: 9 in, 1 out]
            "Exp 10" <- TRUE
            "Temp 3" <- w240
            "Flow 3" <- w239
            "Conc 3" <- w238
          }
          frame 5 {
            n66 = flat-sequence {
              tunnel: w290 -> [w298]
              tunnel: w289 -> [w291]
              tunnel: w289 -> [w362]
              tunnel: w287 -> [w342]
              tunnel: w286 -> [w341]
              tunnel: [w325] -> w285
              tunnel: [w324] -> w284
              tunnel: [w323] -> w283
              tunnel: w282 -> [w313]
              frame #0 {
                # "make this include a write to record file step"
                n67 = call <vilib>:"New Session.vi"("Path to Python Module (.py File)"=path "C:/Users/User/Documents/LabVIEW Data/2015 Projects/Combined/HPLCandAppend.py") -> ("error out"=w309:errorcluster, "Session ID out"=w308:T4)  [unwired: 9 in]
                n68 = call <vilib>:"Pack.vi"("Argument"=w298, "error in (no error)"=w309, "Session ID"=w308) -> ("error out"=w293:errorcluster, "Python Object References Out"=w295:T5, "Session ID out"=w297:T4)  [unwired: 6 in]
                n69 = call <vilib>:"Pack.vi"("Argument"=w291, "error in (no error)"=w293, "Python Object References In"=w295, "Session ID"=w297) -> ("error out"=w292:errorcluster, "Python Object References Out"=w294:T5, "Session ID out"=w296:T4)  [unwired: 5 in]
                n70 = call <vilib>:"Call.vi"("Function or Method Name"="HPLC", "error in (no error)"=w292, "Python Object References In"=w294, "Session ID"=w296) -> ("error out"=w310:errorcluster, "Python Object References Out"=w301:T5, "Session ID out"=w302:T4)  [unwired: 5 in]
                n71 = call-poly <vilib>:"Unpack.vi"("error in (no error)"=w310, "Python Object References In"=w301, "Session ID"=w302) -> ("error out"=w311:errorcluster, "Value"=→"C BAcid 3":dbl, "Python Object References Out"=w306:T5, "Session ID out"=w305:T4)  [unwired: 5 in]
                n72 = call-poly <vilib>:"Unpack.vi"("error in (no error)"=w311, "Python Object References In"=w306, "Session ID"=w305) -> ("error out"=w312:errorcluster, "Value"=→"C EB 3":dbl, "Session ID out"=w307:T4)  [unwired: 5 in, 1 out]
                n73 = call <vilib>:"Close Session.vi"("error in (no error)"=w312, "Session ID"=w307) -> ()  [unwired: 9 in, 1 out]
              }
              frame #1 {
                # "Number read"
                n74 = call <vilib>:"New Session.vi"("Path to Python Module (.py File)"=path "C:/Users/User/Documents/LabVIEW Data/2015 Projects/Combined/closed_loop_benzoic_acid.py") -> ("error out"=w367:errorcluster, "Session ID out"=w366:T4)  [unwired: 9 in]
                n75 = call <vilib>:"Pack.vi"("Argument"=w362, "error in (no error)"=w367, "Session ID"=w366) -> ("error out"=w344:errorcluster, "Python Object References Out"=w346:T5, "Session ID out"=w348:T4)  [unwired: 6 in]
                n76 = call <vilib>:"Pack.vi"("Argument"=w342, "error in (no error)"=w344, "Python Object References In"=w346, "Session ID"=w348) -> ("error out"=w343:errorcluster, "Python Object References Out"=w345:T5, "Session ID out"=w347:T4)  [unwired: 5 in]
                n77 = call <vilib>:"Pack.vi"("Argument"=w341, "error in (no error)"=w343, "Python Object References In"=w345, "Session ID"=w347) -> ("error out"=w315:errorcluster, "Python Object References Out"=w317:T5, "Session ID out"=w319:T4)  [unwired: 5 in]
                n78 = call <vilib>:"Pack.vi"("Argument"=w313, "error in (no error)"=w315, "Python Object References In"=w317, "Session ID"=w319) -> ("error out"=w314:errorcluster, "Python Object References Out"=w316:T5, "Session ID out"=w318:T4)  [unwired: 5 in]
                n79 = call <vilib>:"Call.vi"("Function or Method Name"="design_next_experiment", "error in (no error)"=w314, "Python Object References In"=w316, "Session ID"=w318) -> ("error out"=w328:errorcluster, "Python Object References Out"=w331:T5, "Session ID out"=w334:T4)  [unwired: 5 in]
                n80 = call-poly <vilib>:"Unpack.vi"("error in (no error)"=w328, "Python Object References In"=w331, "Session ID"=w334) -> ("error out"=w327:errorcluster, "Value"=w323:dbl, "Python Object References Out"=w330:T5, "Session ID out"=w333:T4)  [unwired: 5 in]
                "Temp 4" <- w323
                n81 = call-poly <vilib>:"Unpack.vi"("error in (no error)"=w327, "Python Object References In"=w330, "Session ID"=w333) -> ("error out"=w326:errorcluster, "Value"=w324:dbl, "Python Object References Out"=w329:T5, "Session ID out"=w332:T4)  [unwired: 5 in]
                "Flow 4" <- w324
                n82 = call-poly <vilib>:"Unpack.vi"("error in (no error)"=w326, "Python Object References In"=w329, "Session ID"=w332) -> ("error out"=w320:errorcluster, "Value"=w325:dbl, "Python Object References Out"=w321:T5, "Session ID out"=w322:T4)  [unwired: 5 in]
                "Conc 4" <- w325
                n83 = call-poly <vilib>:"Unpack.vi"("error in (no error)"=w320, "Python Object References In"=w321, "Session ID"=w322) -> ("error out"=w372:errorcluster, "Value"=→"Param 1 3":dbl, "Python Object References Out"=w370:T5, "Session ID out"=w368:T4)  [unwired: 5 in]
                n84 = call-poly <vilib>:"Unpack.vi"("error in (no error)"=w372, "Python Object References In"=w370, "Session ID"=w368) -> ("error out"=w373:errorcluster, "Value"=→"T value 1 3":dbl, "Python Object References Out"=w371:T5, "Session ID out"=w369:T4)  [unwired: 5 in]
                n85 = call-poly <vilib>:"Unpack.vi"("error in (no error)"=w373, "Python Object References In"=w371, "Session ID"=w369) -> ("error out"=w374:errorcluster, "Value"=→"Param 2 3":dbl, "Python Object References Out"=w365:T5, "Session ID out"=w364:T4)  [unwired: 5 in]
                n86 = call-poly <vilib>:"Unpack.vi"("error in (no error)"=w374, "Python Object References In"=w365, "Session ID"=w364) -> ("error out"=w356:errorcluster, "Value"=→"T value 2 3":dbl, "Python Object References Out"=w358:T5, "Session ID out"=w360:T4)  [unwired: 5 in]
                n87 = call-poly <vilib>:"Unpack.vi"("error in (no error)"=w356, "Python Object References In"=w358, "Session ID"=w360) -> ("error out"=w355:errorcluster, "Value"=→"T Ref 3":dbl, "Python Object References Out"=w357:T5, "Session ID out"=w359:T4)  [unwired: 5 in]
                n88 = call-poly <vilib>:"Unpack.vi"("error in (no error)"=w355, "Python Object References In"=w357, "Session ID"=w359) -> ("error out"=w338:errorcluster, "Value"=→"Correlation 3":dbl, "Python Object References Out"=w339:T5, "Session ID out"=w340:T4)  [unwired: 5 in]
                n89 = call-poly <vilib>:"Unpack.vi"("error in (no error)"=w338, "Python Object References In"=w339, "Session ID"=w340) -> ("error out"=w352:errorcluster, "Value"=→"X2 3":dbl, "Python Object References Out"=w351:T5, "Session ID out"=w350:T4)  [unwired: 5 in]
                n90 = call-poly <vilib>:"Unpack.vi"("error in (no error)"=w352, "Python Object References In"=w351, "Session ID"=w350) -> ("error out"=w335:errorcluster, "Value"=→"X2 ref 3":dbl, "Session ID out"=w336:T4)  [unwired: 5 in, 1 out]
                n91 = call <vilib>:"Close Session.vi"("error in (no error)"=w335, "Session ID"=w336) -> ()  [unwired: 9 in, 1 out]
              }
            }
            "Exp 4" <- TRUE
          }
          frame 6 {
            n92 = flat-sequence {
              tunnel: w387 -> [w395]
              tunnel: w386 -> [w388]
              tunnel: w386 -> [w459]
              tunnel: w384 -> [w439]
              tunnel: w383 -> [w438]
              tunnel: [w422] -> w382
              tunnel: [w421] -> w381
              tunnel: [w420] -> w380
              tunnel: w379 -> [w410]
              frame #0 {
                # "make this include a write to record file step"
                n93 = call <vilib>:"New Session.vi"("Path to Python Module (.py File)"=path "C:/Users/User/Documents/LabVIEW Data/2015 Projects/Combined/HPLCandAppend.py") -> ("error out"=w406:errorcluster, "Session ID out"=w405:T4)  [unwired: 9 in]
                n94 = call <vilib>:"Pack.vi"("Argument"=w395, "error in (no error)"=w406, "Session ID"=w405) -> ("error out"=w390:errorcluster, "Python Object References Out"=w392:T5, "Session ID out"=w394:T4)  [unwired: 6 in]
                n95 = call <vilib>:"Pack.vi"("Argument"=w388, "error in (no error)"=w390, "Python Object References In"=w392, "Session ID"=w394) -> ("error out"=w389:errorcluster, "Python Object References Out"=w391:T5, "Session ID out"=w393:T4)  [unwired: 5 in]
                n96 = call <vilib>:"Call.vi"("Function or Method Name"="HPLC", "error in (no error)"=w389, "Python Object References In"=w391, "Session ID"=w393) -> ("error out"=w407:errorcluster, "Python Object References Out"=w398:T5, "Session ID out"=w399:T4)  [unwired: 5 in]
                n97 = call-poly <vilib>:"Unpack.vi"("error in (no error)"=w407, "Python Object References In"=w398, "Session ID"=w399) -> ("error out"=w408:errorcluster, "Value"=→"C BAcid 4":dbl, "Python Object References Out"=w403:T5, "Session ID out"=w402:T4)  [unwired: 5 in]
                n98 = call-poly <vilib>:"Unpack.vi"("error in (no error)"=w408, "Python Object References In"=w403, "Session ID"=w402) -> ("error out"=w409:errorcluster, "Value"=→"C EB 4":dbl, "Session ID out"=w404:T4)  [unwired: 5 in, 1 out]
                n99 = call <vilib>:"Close Session.vi"("error in (no error)"=w409, "Session ID"=w404) -> ()  [unwired: 9 in, 1 out]
              }
              frame #1 {
                # "Number read"
                n100 = call <vilib>:"New Session.vi"("Path to Python Module (.py File)"=path "C:/Users/User/Documents/LabVIEW Data/2015 Projects/Combined/closed_loop_benzoic_acid.py") -> ("error out"=w464:errorcluster, "Session ID out"=w463:T4)  [unwired: 9 in]
                n101 = call <vilib>:"Pack.vi"("Argument"=w459, "error in (no error)"=w464, "Session ID"=w463) -> ("error out"=w441:errorcluster, "Python Object References Out"=w443:T5, "Session ID out"=w445:T4)  [unwired: 6 in]
                n102 = call <vilib>:"Pack.vi"("Argument"=w439, "error in (no error)"=w441, "Python Object References In"=w443, "Session ID"=w445) -> ("error out"=w440:errorcluster, "Python Object References Out"=w442:T5, "Session ID out"=w444:T4)  [unwired: 5 in]
                n103 = call <vilib>:"Pack.vi"("Argument"=w438, "error in (no error)"=w440, "Python Object References In"=w442, "Session ID"=w444) -> ("error out"=w412:errorcluster, "Python Object References Out"=w413:T5, "Session ID out"=w416:T4)  [unwired: 5 in]
                n104 = call <vilib>:"Pack.vi"("Argument"=w410, "error in (no error)"=w412, "Python Object References In"=w413, "Session ID"=w416) -> ("error out"=w411:errorcluster, "Python Object References Out"=w414:T5, "Session ID out"=w415:T4)  [unwired: 5 in]
                n105 = call <vilib>:"Call.vi"("Function or Method Name"="design_next_experiment", "error in (no error)"=w411, "Python Object References In"=w414, "Session ID"=w415) -> ("error out"=w425:errorcluster, "Python Object References Out"=w428:T5, "Session ID out"=w431:T4)  [unwired: 5 in]
                n106 = call-poly <vilib>:"Unpack.vi"("error in (no error)"=w425, "Python Object References In"=w428, "Session ID"=w431) -> ("error out"=w424:errorcluster, "Value"=w420:dbl, "Python Object References Out"=w427:T5, "Session ID out"=w430:T4)  [unwired: 5 in]
                "Temp 5" <- w420
                n107 = call-poly <vilib>:"Unpack.vi"("error in (no error)"=w424, "Python Object References In"=w427, "Session ID"=w430) -> ("error out"=w423:errorcluster, "Value"=w421:dbl, "Python Object References Out"=w426:T5, "Session ID out"=w429:T4)  [unwired: 5 in]
                "Flow 5" <- w421
                n108 = call-poly <vilib>:"Unpack.vi"("error in (no error)"=w423, "Python Object References In"=w426, "Session ID"=w429) -> ("error out"=w417:errorcluster, "Value"=w422:dbl, "Python Object References Out"=w418:T5, "Session ID out"=w419:T4)  [unwired: 5 in]
                "Conc 5" <- w422
                n109 = call-poly <vilib>:"Unpack.vi"("error in (no error)"=w417, "Python Object References In"=w418, "Session ID"=w419) -> ("error out"=w469:errorcluster, "Value"=→"Param 1 4":dbl, "Python Object References Out"=w467:T5, "Session ID out"=w465:T4)  [unwired: 5 in]
                n110 = call-poly <vilib>:"Unpack.vi"("error in (no error)"=w469, "Python Object References In"=w467, "Session ID"=w465) -> ("error out"=w470:errorcluster, "Value"=→"T value 1 4":dbl, "Python Object References Out"=w468:T5, "Session ID out"=w466:T4)  [unwired: 5 in]
                n111 = call-poly <vilib>:"Unpack.vi"("error in (no error)"=w470, "Python Object References In"=w468, "Session ID"=w466) -> ("error out"=w471:errorcluster, "Value"=→"Param 2 4":dbl, "Python Object References Out"=w462:T5, "Session ID out"=w461:T4)  [unwired: 5 in]
                n112 = call-poly <vilib>:"Unpack.vi"("error in (no error)"=w471, "Python Object References In"=w462, "Session ID"=w461) -> ("error out"=w453:errorcluster, "Value"=→"T value 2 4":dbl, "Python Object References Out"=w455:T5, "Session ID out"=w457:T4)  [unwired: 5 in]
                n113 = call-poly <vilib>:"Unpack.vi"("error in (no error)"=w453, "Python Object References In"=w455, "Session ID"=w457) -> ("error out"=w452:errorcluster, "Value"=→"T Ref 4":dbl, "Python Object References Out"=w454:T5, "Session ID out"=w456:T4)  [unwired: 5 in]
                n114 = call-poly <vilib>:"Unpack.vi"("error in (no error)"=w452, "Python Object References In"=w454, "Session ID"=w456) -> ("error out"=w435:errorcluster, "Value"=→"Correlation 4":dbl, "Python Object References Out"=w436:T5, "Session ID out"=w437:T4)  [unwired: 5 in]
                n115 = call-poly <vilib>:"Unpack.vi"("error in (no error)"=w435, "Python Object References In"=w436, "Session ID"=w437) -> ("error out"=w449:errorcluster, "Value"=→"X2 4":dbl, "Python Object References Out"=w448:T5, "Session ID out"=w447:T4)  [unwired: 5 in]
                n116 = call-poly <vilib>:"Unpack.vi"("error in (no error)"=w449, "Python Object References In"=w448, "Session ID"=w447) -> ("error out"=w432:errorcluster, "Value"=→"X2 ref 4":dbl, "Session ID out"=w433:T4)  [unwired: 5 in, 1 out]
                n117 = call <vilib>:"Close Session.vi"("error in (no error)"=w432, "Session ID"=w433) -> ()  [unwired: 9 in, 1 out]
              }
            }
            "Exp 5" <- TRUE
          }
          frame 7 {
            n118 = flat-sequence {
              tunnel: w484 -> [w492]
              tunnel: w483 -> [w485]
              tunnel: w483 -> [w556]
              tunnel: w481 -> [w536]
              tunnel: w480 -> [w535]
              tunnel: [w519] -> w479
              tunnel: [w518] -> w478
              tunnel: [w517] -> w477
              tunnel: w476 -> [w507]
              frame #0 {
                # "make this include a write to record file step"
                n119 = call <vilib>:"New Session.vi"("Path to Python Module (.py File)"=path "C:/Users/User/Documents/LabVIEW Data/2015 Projects/Combined/HPLCandAppend.py") -> ("error out"=w503:errorcluster, "Session ID out"=w502:T4)  [unwired: 9 in]
                n120 = call <vilib>:"Pack.vi"("Argument"=w492, "error in (no error)"=w503, "Session ID"=w502) -> ("error out"=w487:errorcluster, "Python Object References Out"=w489:T5, "Session ID out"=w491:T4)  [unwired: 6 in]
                n121 = call <vilib>:"Pack.vi"("Argument"=w485, "error in (no error)"=w487, "Python Object References In"=w489, "Session ID"=w491) -> ("error out"=w486:errorcluster, "Python Object References Out"=w488:T5, "Session ID out"=w490:T4)  [unwired: 5 in]
                n122 = call <vilib>:"Call.vi"("Function or Method Name"="HPLC", "error in (no error)"=w486, "Python Object References In"=w488, "Session ID"=w490) -> ("error out"=w504:errorcluster, "Python Object References Out"=w495:T5, "Session ID out"=w496:T4)  [unwired: 5 in]
                n123 = call-poly <vilib>:"Unpack.vi"("error in (no error)"=w504, "Python Object References In"=w495, "Session ID"=w496) -> ("error out"=w505:errorcluster, "Value"=→"C BAcid 5":dbl, "Python Object References Out"=w500:T5, "Session ID out"=w499:T4)  [unwired: 5 in]
                n124 = call-poly <vilib>:"Unpack.vi"("error in (no error)"=w505, "Python Object References In"=w500, "Session ID"=w499) -> ("error out"=w506:errorcluster, "Value"=→"C EB 5":dbl, "Session ID out"=w501:T4)  [unwired: 5 in, 1 out]
                n125 = call <vilib>:"Close Session.vi"("error in (no error)"=w506, "Session ID"=w501) -> ()  [unwired: 9 in, 1 out]
              }
              frame #1 {
                # "Number read"
                n126 = call <vilib>:"New Session.vi"("Path to Python Module (.py File)"=path "C:/Users/User/Documents/LabVIEW Data/2015 Projects/Combined/closed_loop_benzoic_acid.py") -> ("error out"=w561:errorcluster, "Session ID out"=w560:T4)  [unwired: 9 in]
                n127 = call <vilib>:"Pack.vi"("Argument"=w556, "error in (no error)"=w561, "Session ID"=w560) -> ("error out"=w538:errorcluster, "Python Object References Out"=w540:T5, "Session ID out"=w542:T4)  [unwired: 6 in]
                n128 = call <vilib>:"Pack.vi"("Argument"=w536, "error in (no error)"=w538, "Python Object References In"=w540, "Session ID"=w542) -> ("error out"=w537:errorcluster, "Python Object References Out"=w539:T5, "Session ID out"=w541:T4)  [unwired: 5 in]
                n129 = call <vilib>:"Pack.vi"("Argument"=w535, "error in (no error)"=w537, "Python Object References In"=w539, "Session ID"=w541) -> ("error out"=w508:errorcluster, "Python Object References Out"=w511:T5, "Session ID out"=w513:T4)  [unwired: 5 in]
                n130 = call <vilib>:"Pack.vi"("Argument"=w507, "error in (no error)"=w508, "Python Object References In"=w511, "Session ID"=w513) -> ("error out"=w509:errorcluster, "Python Object References Out"=w510:T5, "Session ID out"=w512:T4)  [unwired: 5 in]
                n131 = call <vilib>:"Call.vi"("Function or Method Name"="design_next_experiment", "error in (no error)"=w509, "Python Object References In"=w510, "Session ID"=w512) -> ("error out"=w522:errorcluster, "Python Object References Out"=w525:T5, "Session ID out"=w528:T4)  [unwired: 5 in]
                n132 = call-poly <vilib>:"Unpack.vi"("error in (no error)"=w522, "Python Object References In"=w525, "Session ID"=w528) -> ("error out"=w521:errorcluster, "Value"=w517:dbl, "Python Object References Out"=w524:T5, "Session ID out"=w527:T4)  [unwired: 5 in]
                "Temp 6" <- w517
                n133 = call-poly <vilib>:"Unpack.vi"("error in (no error)"=w521, "Python Object References In"=w524, "Session ID"=w527) -> ("error out"=w520:errorcluster, "Value"=w518:dbl, "Python Object References Out"=w523:T5, "Session ID out"=w526:T4)  [unwired: 5 in]
                "Flow 6" <- w518
                n134 = call-poly <vilib>:"Unpack.vi"("error in (no error)"=w520, "Python Object References In"=w523, "Session ID"=w526) -> ("error out"=w514:errorcluster, "Value"=w519:dbl, "Python Object References Out"=w515:T5, "Session ID out"=w516:T4)  [unwired: 5 in]
                "Conc 6" <- w519
                n135 = call-poly <vilib>:"Unpack.vi"("error in (no error)"=w514, "Python Object References In"=w515, "Session ID"=w516) -> ("error out"=w566:errorcluster, "Value"=→"Param 1 5":dbl, "Python Object References Out"=w564:T5, "Session ID out"=w562:T4)  [unwired: 5 in]
                n136 = call-poly <vilib>:"Unpack.vi"("error in (no error)"=w566, "Python Object References In"=w564, "Session ID"=w562) -> ("error out"=w567:errorcluster, "Value"=→"T value 1 5":dbl, "Python Object References Out"=w565:T5, "Session ID out"=w563:T4)  [unwired: 5 in]
                n137 = call-poly <vilib>:"Unpack.vi"("error in (no error)"=w567, "Python Object References In"=w565, "Session ID"=w563) -> ("error out"=w568:errorcluster, "Value"=→"Param 2 5":dbl, "Python Object References Out"=w559:T5, "Session ID out"=w558:T4)  [unwired: 5 in]
                n138 = call-poly <vilib>:"Unpack.vi"("error in (no error)"=w568, "Python Object References In"=w559, "Session ID"=w558) -> ("error out"=w550:errorcluster, "Value"=→"T value 2 5":dbl, "Python Object References Out"=w552:T5, "Session ID out"=w554:T4)  [unwired: 5 in]
                n139 = call-poly <vilib>:"Unpack.vi"("error in (no error)"=w550, "Python Object References In"=w552, "Session ID"=w554) -> ("error out"=w549:errorcluster, "Value"=→"T Ref 5":dbl, "Python Object References Out"=w551:T5, "Session ID out"=w553:T4)  [unwired: 5 in]
                n140 = call-poly <vilib>:"Unpack.vi"("error in (no error)"=w549, "Python Object References In"=w551, "Session ID"=w553) -> ("error out"=w532:errorcluster, "Value"=→"Correlation 5":dbl, "Python Object References Out"=w533:T5, "Session ID out"=w534:T4)  [unwired: 5 in]
                n141 = call-poly <vilib>:"Unpack.vi"("error in (no error)"=w532, "Python Object References In"=w533, "Session ID"=w534) -> ("error out"=w546:errorcluster, "Value"=→"X2 5":dbl, "Python Object References Out"=w545:T5, "Session ID out"=w544:T4)  [unwired: 5 in]
                n142 = call-poly <vilib>:"Unpack.vi"("error in (no error)"=w546, "Python Object References In"=w545, "Session ID"=w544) -> ("error out"=w529:errorcluster, "Value"=→"X2 ref 5":dbl, "Session ID out"=w530:T4)  [unwired: 5 in, 1 out]
                n143 = call <vilib>:"Close Session.vi"("error in (no error)"=w529, "Session ID"=w530) -> ()  [unwired: 9 in, 1 out]
              }
            }
            "Exp 6" <- TRUE
          }
          frame 8 {
            n144 = flat-sequence {
              tunnel: w581 -> [w589]
              tunnel: w580 -> [w582]
              tunnel: w580 -> [w653]
              tunnel: w578 -> [w633]
              tunnel: w577 -> [w632]
              tunnel: [w616] -> w576
              tunnel: [w615] -> w575
              tunnel: [w614] -> w574
              tunnel: w573 -> [w604]
              frame #0 {
                # "make this include a write to record file step"
                n145 = call <vilib>:"New Session.vi"("Path to Python Module (.py File)"=path "C:/Users/User/Documents/LabVIEW Data/2015 Projects/Combined/HPLCandAppend.py") -> ("error out"=w600:errorcluster, "Session ID out"=w599:T4)  [unwired: 9 in]
                n146 = call <vilib>:"Pack.vi"("Argument"=w589, "error in (no error)"=w600, "Session ID"=w599) -> ("error out"=w584:errorcluster, "Python Object References Out"=w586:T5, "Session ID out"=w588:T4)  [unwired: 6 in]
                n147 = call <vilib>:"Pack.vi"("Argument"=w582, "error in (no error)"=w584, "Python Object References In"=w586, "Session ID"=w588) -> ("error out"=w583:errorcluster, "Python Object References Out"=w585:T5, "Session ID out"=w587:T4)  [unwired: 5 in]
                n148 = call <vilib>:"Call.vi"("Function or Method Name"="HPLC", "error in (no error)"=w583, "Python Object References In"=w585, "Session ID"=w587) -> ("error out"=w601:errorcluster, "Python Object References Out"=w592:T5, "Session ID out"=w593:T4)  [unwired: 5 in]
                n149 = call-poly <vilib>:"Unpack.vi"("error in (no error)"=w601, "Python Object References In"=w592, "Session ID"=w593) -> ("error out"=w602:errorcluster, "Value"=→"C BAcid 6":dbl, "Python Object References Out"=w597:T5, "Session ID out"=w596:T4)  [unwired: 5 in]
                n150 = call-poly <vilib>:"Unpack.vi"("error in (no error)"=w602, "Python Object References In"=w597, "Session ID"=w596) -> ("error out"=w603:errorcluster, "Value"=→"C EB 6":dbl, "Session ID out"=w598:T4)  [unwired: 5 in, 1 out]
                n151 = call <vilib>:"Close Session.vi"("error in (no error)"=w603, "Session ID"=w598) -> ()  [unwired: 9 in, 1 out]
              }
              frame #1 {
                # "Number read"
                n152 = call <vilib>:"New Session.vi"("Path to Python Module (.py File)"=path "C:/Users/User/Documents/LabVIEW Data/2015 Projects/Combined/closed_loop_benzoic_acid.py") -> ("error out"=w658:errorcluster, "Session ID out"=w657:T4)  [unwired: 9 in]
                n153 = call <vilib>:"Pack.vi"("Argument"=w653, "error in (no error)"=w658, "Session ID"=w657) -> ("error out"=w635:errorcluster, "Python Object References Out"=w637:T5, "Session ID out"=w639:T4)  [unwired: 6 in]
                n154 = call <vilib>:"Pack.vi"("Argument"=w633, "error in (no error)"=w635, "Python Object References In"=w637, "Session ID"=w639) -> ("error out"=w634:errorcluster, "Python Object References Out"=w636:T5, "Session ID out"=w638:T4)  [unwired: 5 in]
                n155 = call <vilib>:"Pack.vi"("Argument"=w632, "error in (no error)"=w634, "Python Object References In"=w636, "Session ID"=w638) -> ("error out"=w605:errorcluster, "Python Object References Out"=w608:T5, "Session ID out"=w610:T4)  [unwired: 5 in]
                n156 = call <vilib>:"Pack.vi"("Argument"=w604, "error in (no error)"=w605, "Python Object References In"=w608, "Session ID"=w610) -> ("error out"=w606:errorcluster, "Python Object References Out"=w607:T5, "Session ID out"=w609:T4)  [unwired: 5 in]
                n157 = call <vilib>:"Call.vi"("Function or Method Name"="design_next_experiment", "error in (no error)"=w606, "Python Object References In"=w607, "Session ID"=w609) -> ("error out"=w619:errorcluster, "Python Object References Out"=w622:T5, "Session ID out"=w625:T4)  [unwired: 5 in]
                n158 = call-poly <vilib>:"Unpack.vi"("error in (no error)"=w619, "Python Object References In"=w622, "Session ID"=w625) -> ("error out"=w618:errorcluster, "Value"=w614:dbl, "Python Object References Out"=w621:T5, "Session ID out"=w624:T4)  [unwired: 5 in]
                "Temp 7" <- w614
                n159 = call-poly <vilib>:"Unpack.vi"("error in (no error)"=w618, "Python Object References In"=w621, "Session ID"=w624) -> ("error out"=w617:errorcluster, "Value"=w615:dbl, "Python Object References Out"=w620:T5, "Session ID out"=w623:T4)  [unwired: 5 in]
                "Flow 7" <- w615
                n160 = call-poly <vilib>:"Unpack.vi"("error in (no error)"=w617, "Python Object References In"=w620, "Session ID"=w623) -> ("error out"=w611:errorcluster, "Value"=w616:dbl, "Python Object References Out"=w612:T5, "Session ID out"=w613:T4)  [unwired: 5 in]
                "Conc 7" <- w616
                n161 = call-poly <vilib>:"Unpack.vi"("error in (no error)"=w611, "Python Object References In"=w612, "Session ID"=w613) -> ("error out"=w663:errorcluster, "Value"=→"Param 1 6":dbl, "Python Object References Out"=w661:T5, "Session ID out"=w659:T4)  [unwired: 5 in]
                n162 = call-poly <vilib>:"Unpack.vi"("error in (no error)"=w663, "Python Object References In"=w661, "Session ID"=w659) -> ("error out"=w664:errorcluster, "Value"=→"T value 1 6":dbl, "Python Object References Out"=w662:T5, "Session ID out"=w660:T4)  [unwired: 5 in]
                n163 = call-poly <vilib>:"Unpack.vi"("error in (no error)"=w664, "Python Object References In"=w662, "Session ID"=w660) -> ("error out"=w665:errorcluster, "Value"=→"Param 2 6":dbl, "Python Object References Out"=w656:T5, "Session ID out"=w655:T4)  [unwired: 5 in]
                n164 = call-poly <vilib>:"Unpack.vi"("error in (no error)"=w665, "Python Object References In"=w656, "Session ID"=w655) -> ("error out"=w647:errorcluster, "Value"=→"T value 2 6":dbl, "Python Object References Out"=w649:T5, "Session ID out"=w651:T4)  [unwired: 5 in]
                n165 = call-poly <vilib>:"Unpack.vi"("error in (no error)"=w647, "Python Object References In"=w649, "Session ID"=w651) -> ("error out"=w646:errorcluster, "Value"=→"T Ref 6":dbl, "Python Object References Out"=w648:T5, "Session ID out"=w650:T4)  [unwired: 5 in]
                n166 = call-poly <vilib>:"Unpack.vi"("error in (no error)"=w646, "Python Object References In"=w648, "Session ID"=w650) -> ("error out"=w629:errorcluster, "Value"=→"Correlation 6":dbl, "Python Object References Out"=w630:T5, "Session ID out"=w631:T4)  [unwired: 5 in]
                n167 = call-poly <vilib>:"Unpack.vi"("error in (no error)"=w629, "Python Object References In"=w630, "Session ID"=w631) -> ("error out"=w643:errorcluster, "Value"=→"X2 6":dbl, "Python Object References Out"=w642:T5, "Session ID out"=w641:T4)  [unwired: 5 in]
                n168 = call-poly <vilib>:"Unpack.vi"("error in (no error)"=w643, "Python Object References In"=w642, "Session ID"=w641) -> ("error out"=w626:errorcluster, "Value"=→"X2 ref 6":dbl, "Session ID out"=w627:T4)  [unwired: 5 in, 1 out]
                n169 = call <vilib>:"Close Session.vi"("error in (no error)"=w626, "Session ID"=w627) -> ()  [unwired: 9 in, 1 out]
              }
            }
            "Exp 7" <- TRUE
          }
          frame 9 {
            n170 = flat-sequence {
              tunnel: w678 -> [w686]
              tunnel: w677 -> [w679]
              tunnel: w677 -> [w750]
              tunnel: w675 -> [w730]
              tunnel: w674 -> [w729]
              tunnel: [w713] -> w673
              tunnel: [w712] -> w672
              tunnel: [w711] -> w671
              tunnel: w670 -> [w701]
              frame #0 {
                # "make this include a write to record file step"
                n171 = call <vilib>:"New Session.vi"("Path to Python Module (.py File)"=path "C:/Users/User/Documents/LabVIEW Data/2015 Projects/Combined/HPLCandAppend.py") -> ("error out"=w697:errorcluster, "Session ID out"=w696:T4)  [unwired: 9 in]
                n172 = call <vilib>:"Pack.vi"("Argument"=w686, "error in (no error)"=w697, "Session ID"=w696) -> ("error out"=w681:errorcluster, "Python Object References Out"=w683:T5, "Session ID out"=w685:T4)  [unwired: 6 in]
                n173 = call <vilib>:"Pack.vi"("Argument"=w679, "error in (no error)"=w681, "Python Object References In"=w683, "Session ID"=w685) -> ("error out"=w680:errorcluster, "Python Object References Out"=w682:T5, "Session ID out"=w684:T4)  [unwired: 5 in]
                n174 = call <vilib>:"Call.vi"("Function or Method Name"="HPLC", "error in (no error)"=w680, "Python Object References In"=w682, "Session ID"=w684) -> ("error out"=w698:errorcluster, "Python Object References Out"=w689:T5, "Session ID out"=w690:T4)  [unwired: 5 in]
                n175 = call-poly <vilib>:"Unpack.vi"("error in (no error)"=w698, "Python Object References In"=w689, "Session ID"=w690) -> ("error out"=w699:errorcluster, "Value"=→"C BAcid 7":dbl, "Python Object References Out"=w694:T5, "Session ID out"=w693:T4)  [unwired: 5 in]
                n176 = call-poly <vilib>:"Unpack.vi"("error in (no error)"=w699, "Python Object References In"=w694, "Session ID"=w693) -> ("error out"=w700:errorcluster, "Value"=→"C EB 7":dbl, "Session ID out"=w695:T4)  [unwired: 5 in, 1 out]
                n177 = call <vilib>:"Close Session.vi"("error in (no error)"=w700, "Session ID"=w695) -> ()  [unwired: 9 in, 1 out]
              }
              frame #1 {
                # "Number read"
                n178 = call <vilib>:"New Session.vi"("Path to Python Module (.py File)"=path "C:/Users/User/Documents/LabVIEW Data/2015 Projects/Combined/closed_loop_benzoic_acid.py") -> ("error out"=w755:errorcluster, "Session ID out"=w754:T4)  [unwired: 9 in]
                n179 = call <vilib>:"Pack.vi"("Argument"=w750, "error in (no error)"=w755, "Session ID"=w754) -> ("error out"=w732:errorcluster, "Python Object References Out"=w734:T5, "Session ID out"=w736:T4)  [unwired: 6 in]
                n180 = call <vilib>:"Pack.vi"("Argument"=w730, "error in (no error)"=w732, "Python Object References In"=w734, "Session ID"=w736) -> ("error out"=w731:errorcluster, "Python Object References Out"=w733:T5, "Session ID out"=w735:T4)  [unwired: 5 in]
                n181 = call <vilib>:"Pack.vi"("Argument"=w729, "error in (no error)"=w731, "Python Object References In"=w733, "Session ID"=w735) -> ("error out"=w703:errorcluster, "Python Object References Out"=w705:T5, "Session ID out"=w707:T4)  [unwired: 5 in]
                n182 = call <vilib>:"Pack.vi"("Argument"=w701, "error in (no error)"=w703, "Python Object References In"=w705, "Session ID"=w707) -> ("error out"=w702:errorcluster, "Python Object References Out"=w704:T5, "Session ID out"=w706:T4)  [unwired: 5 in]
                n183 = call <vilib>:"Call.vi"("Function or Method Name"="design_next_experiment", "error in (no error)"=w702, "Python Object References In"=w704, "Session ID"=w706) -> ("error out"=w716:errorcluster, "Python Object References Out"=w719:T5, "Session ID out"=w722:T4)  [unwired: 5 in]
                n184 = call-poly <vilib>:"Unpack.vi"("error in (no error)"=w716, "Python Object References In"=w719, "Session ID"=w722) -> ("error out"=w715:errorcluster, "Value"=w711:dbl, "Python Object References Out"=w718:T5, "Session ID out"=w721:T4)  [unwired: 5 in]
                "Temp 8" <- w711
                n185 = call-poly <vilib>:"Unpack.vi"("error in (no error)"=w715, "Python Object References In"=w718, "Session ID"=w721) -> ("error out"=w714:errorcluster, "Value"=w712:dbl, "Python Object References Out"=w717:T5, "Session ID out"=w720:T4)  [unwired: 5 in]
                "Flow 8" <- w712
                n186 = call-poly <vilib>:"Unpack.vi"("error in (no error)"=w714, "Python Object References In"=w717, "Session ID"=w720) -> ("error out"=w708:errorcluster, "Value"=w713:dbl, "Python Object References Out"=w709:T5, "Session ID out"=w710:T4)  [unwired: 5 in]
                "Conc 8" <- w713
                n187 = call-poly <vilib>:"Unpack.vi"("error in (no error)"=w708, "Python Object References In"=w709, "Session ID"=w710) -> ("error out"=w760:errorcluster, "Value"=→"Param 1 7":dbl, "Python Object References Out"=w758:T5, "Session ID out"=w756:T4)  [unwired: 5 in]
                n188 = call-poly <vilib>:"Unpack.vi"("error in (no error)"=w760, "Python Object References In"=w758, "Session ID"=w756) -> ("error out"=w761:errorcluster, "Value"=→"T value 1 7":dbl, "Python Object References Out"=w759:T5, "Session ID out"=w757:T4)  [unwired: 5 in]
                n189 = call-poly <vilib>:"Unpack.vi"("error in (no error)"=w761, "Python Object References In"=w759, "Session ID"=w757) -> ("error out"=w762:errorcluster, "Value"=→"Param 2 7":dbl, "Python Object References Out"=w753:T5, "Session ID out"=w752:T4)  [unwired: 5 in]
                n190 = call-poly <vilib>:"Unpack.vi"("error in (no error)"=w762, "Python Object References In"=w753, "Session ID"=w752) -> ("error out"=w744:errorcluster, "Value"=→"T value 2 7":dbl, "Python Object References Out"=w746:T5, "Session ID out"=w748:T4)  [unwired: 5 in]
                n191 = call-poly <vilib>:"Unpack.vi"("error in (no error)"=w744, "Python Object References In"=w746, "Session ID"=w748) -> ("error out"=w743:errorcluster, "Value"=→"T Ref 7":dbl, "Python Object References Out"=w745:T5, "Session ID out"=w747:T4)  [unwired: 5 in]
                n192 = call-poly <vilib>:"Unpack.vi"("error in (no error)"=w743, "Python Object References In"=w745, "Session ID"=w747) -> ("error out"=w726:errorcluster, "Value"=→"Correlation 7":dbl, "Python Object References Out"=w727:T5, "Session ID out"=w728:T4)  [unwired: 5 in]
                n193 = call-poly <vilib>:"Unpack.vi"("error in (no error)"=w726, "Python Object References In"=w727, "Session ID"=w728) -> ("error out"=w740:errorcluster, "Value"=→"X2 7":dbl, "Python Object References Out"=w739:T5, "Session ID out"=w738:T4)  [unwired: 5 in]
                n194 = call-poly <vilib>:"Unpack.vi"("error in (no error)"=w740, "Python Object References In"=w739, "Session ID"=w738) -> ("error out"=w723:errorcluster, "Value"=→"X2 ref 7":dbl, "Session ID out"=w724:T4)  [unwired: 5 in, 1 out]
                n195 = call <vilib>:"Close Session.vi"("error in (no error)"=w723, "Session ID"=w724) -> ()  [unwired: 9 in, 1 out]
              }
            }
            "Exp 8" <- TRUE
          }
          frame 10 {
            n196 = flat-sequence {
              tunnel: w775 -> [w783]
              tunnel: w774 -> [w776]
              tunnel: w774 -> [w847]
              tunnel: w772 -> [w827]
              tunnel: w771 -> [w826]
              tunnel: w770 -> [w801]
              tunnel: [w800] -> w769
              tunnel: [w799] -> w768
              tunnel: [w798] -> w767
              frame #0 {
                # "make this include a write to record file step"
                n197 = call <vilib>:"New Session.vi"("Path to Python Module (.py File)"=path "C:/Users/User/Documents/LabVIEW Data/2015 Projects/Combined/HPLCandAppend.py") -> ("error out"=w794:errorcluster, "Session ID out"=w793:T4)  [unwired: 9 in]
                n198 = call <vilib>:"Pack.vi"("Argument"=w783, "error in (no error)"=w794, "Session ID"=w793) -> ("error out"=w778:errorcluster, "Python Object References Out"=w780:T5, "Session ID out"=w782:T4)  [unwired: 6 in]
                n199 = call <vilib>:"Pack.vi"("Argument"=w776, "error in (no error)"=w778, "Python Object References In"=w780, "Session ID"=w782) -> ("error out"=w777:errorcluster, "Python Object References Out"=w779:T5, "Session ID out"=w781:T4)  [unwired: 5 in]
                n200 = call <vilib>:"Call.vi"("Function or Method Name"="HPLC", "error in (no error)"=w777, "Python Object References In"=w779, "Session ID"=w781) -> ("error out"=w795:errorcluster, "Python Object References Out"=w786:T5, "Session ID out"=w787:T4)  [unwired: 5 in]
                n201 = call-poly <vilib>:"Unpack.vi"("error in (no error)"=w795, "Python Object References In"=w786, "Session ID"=w787) -> ("error out"=w796:errorcluster, "Value"=→"C BAcid 8":dbl, "Python Object References Out"=w791:T5, "Session ID out"=w790:T4)  [unwired: 5 in]
                n202 = call-poly <vilib>:"Unpack.vi"("error in (no error)"=w796, "Python Object References In"=w791, "Session ID"=w790) -> ("error out"=w797:errorcluster, "Value"=→"C EB 8":dbl, "Session ID out"=w792:T4)  [unwired: 5 in, 1 out]
                n203 = call <vilib>:"Close Session.vi"("error in (no error)"=w797, "Session ID"=w792) -> ()  [unwired: 9 in, 1 out]
              }
              frame #1 {
                # "Number read"
                n204 = call <vilib>:"New Session.vi"("Path to Python Module (.py File)"=path "C:/Users/User/Documents/LabVIEW Data/2015 Projects/Combined/closed_loop_benzoic_acid.py") -> ("error out"=w852:errorcluster, "Session ID out"=w851:T4)  [unwired: 9 in]
                n205 = call <vilib>:"Pack.vi"("Argument"=w847, "error in (no error)"=w852, "Session ID"=w851) -> ("error out"=w829:errorcluster, "Python Object References Out"=w831:T5, "Session ID out"=w833:T4)  [unwired: 6 in]
                n206 = call <vilib>:"Pack.vi"("Argument"=w827, "error in (no error)"=w829, "Python Object References In"=w831, "Session ID"=w833) -> ("error out"=w828:errorcluster, "Python Object References Out"=w830:T5, "Session ID out"=w832:T4)  [unwired: 5 in]
                n207 = call <vilib>:"Pack.vi"("Argument"=w826, "error in (no error)"=w828, "Python Object References In"=w830, "Session ID"=w832) -> ("error out"=w803:errorcluster, "Python Object References Out"=w805:T5, "Session ID out"=w807:T4)  [unwired: 5 in]
                n208 = call <vilib>:"Pack.vi"("Argument"=w801, "error in (no error)"=w803, "Python Object References In"=w805, "Session ID"=w807) -> ("error out"=w802:errorcluster, "Python Object References Out"=w804:T5, "Session ID out"=w806:T4)  [unwired: 5 in]
                n209 = call <vilib>:"Call.vi"("Function or Method Name"="design_next_experiment", "error in (no error)"=w802, "Python Object References In"=w804, "Session ID"=w806) -> ("error out"=w813:errorcluster, "Python Object References Out"=w816:T5, "Session ID out"=w819:T4)  [unwired: 5 in]
                n210 = call-poly <vilib>:"Unpack.vi"("error in (no error)"=w813, "Python Object References In"=w816, "Session ID"=w819) -> ("error out"=w812:errorcluster, "Value"=w800:dbl, "Python Object References Out"=w815:T5, "Session ID out"=w818:T4)  [unwired: 5 in]
                "Temp 9" <- w800
                n211 = call-poly <vilib>:"Unpack.vi"("error in (no error)"=w812, "Python Object References In"=w815, "Session ID"=w818) -> ("error out"=w811:errorcluster, "Value"=w799:dbl, "Python Object References Out"=w814:T5, "Session ID out"=w817:T4)  [unwired: 5 in]
                "Flow 9" <- w799
                n212 = call-poly <vilib>:"Unpack.vi"("error in (no error)"=w811, "Python Object References In"=w814, "Session ID"=w817) -> ("error out"=w808:errorcluster, "Value"=w798:dbl, "Python Object References Out"=w809:T5, "Session ID out"=w810:T4)  [unwired: 5 in]
                "Conc 9" <- w798
                n213 = call-poly <vilib>:"Unpack.vi"("error in (no error)"=w808, "Python Object References In"=w809, "Session ID"=w810) -> ("error out"=w857:errorcluster, "Value"=→"Param 1 8":dbl, "Python Object References Out"=w855:T5, "Session ID out"=w853:T4)  [unwired: 5 in]
                n214 = call-poly <vilib>:"Unpack.vi"("error in (no error)"=w857, "Python Object References In"=w855, "Session ID"=w853) -> ("error out"=w858:errorcluster, "Value"=→"T value 1 8":dbl, "Python Object References Out"=w856:T5, "Session ID out"=w854:T4)  [unwired: 5 in]
                n215 = call-poly <vilib>:"Unpack.vi"("error in (no error)"=w858, "Python Object References In"=w856, "Session ID"=w854) -> ("error out"=w859:errorcluster, "Value"=→"Param 2 8":dbl, "Python Object References Out"=w850:T5, "Session ID out"=w849:T4)  [unwired: 5 in]
                n216 = call-poly <vilib>:"Unpack.vi"("error in (no error)"=w859, "Python Object References In"=w850, "Session ID"=w849) -> ("error out"=w841:errorcluster, "Value"=→"T value 2 8":dbl, "Python Object References Out"=w843:T5, "Session ID out"=w845:T4)  [unwired: 5 in]
                n217 = call-poly <vilib>:"Unpack.vi"("error in (no error)"=w841, "Python Object References In"=w843, "Session ID"=w845) -> ("error out"=w840:errorcluster, "Value"=→"T Ref 8":dbl, "Python Object References Out"=w842:T5, "Session ID out"=w844:T4)  [unwired: 5 in]
                n218 = call-poly <vilib>:"Unpack.vi"("error in (no error)"=w840, "Python Object References In"=w842, "Session ID"=w844) -> ("error out"=w823:errorcluster, "Value"=→"Correlation 8":dbl, "Python Object References Out"=w824:T5, "Session ID out"=w825:T4)  [unwired: 5 in]
                n219 = call-poly <vilib>:"Unpack.vi"("error in (no error)"=w823, "Python Object References In"=w824, "Session ID"=w825) -> ("error out"=w837:errorcluster, "Value"=→"X2 8":dbl, "Python Object References Out"=w836:T5, "Session ID out"=w835:T4)  [unwired: 5 in]
                n220 = call-poly <vilib>:"Unpack.vi"("error in (no error)"=w837, "Python Object References In"=w836, "Session ID"=w835) -> ("error out"=w820:errorcluster, "Value"=→"X2 ref 8":dbl, "Session ID out"=w821:T4)  [unwired: 5 in, 1 out]
                n221 = call <vilib>:"Close Session.vi"("error in (no error)"=w820, "Session ID"=w821) -> ()  [unwired: 9 in, 1 out]
              }
            }
            "Exp 9" <- TRUE
          }
          frame 11 {
            n222 = flat-sequence {
              tunnel: w872 -> [w880]
              tunnel: w871 -> [w873]
              tunnel: w871 -> [w944]
              tunnel: w869 -> [w924]
              tunnel: w868 -> [w923]
              tunnel: w867 -> [w895]
              frame #0 {
                # "make this include a write to record file step"
                n223 = call <vilib>:"New Session.vi"("Path to Python Module (.py File)"=path "C:/Users/User/Documents/LabVIEW Data/2015 Projects/Combined/HPLCandAppend.py") -> ("error out"=w891:errorcluster, "Session ID out"=w890:T4)  [unwired: 9 in]
                n224 = call <vilib>:"Pack.vi"("Argument"=w880, "error in (no error)"=w891, "Session ID"=w890) -> ("error out"=w875:errorcluster, "Python Object References Out"=w877:T5, "Session ID out"=w879:T4)  [unwired: 6 in]
                n225 = call <vilib>:"Pack.vi"("Argument"=w873, "error in (no error)"=w875, "Python Object References In"=w877, "Session ID"=w879) -> ("error out"=w874:errorcluster, "Python Object References Out"=w876:T5, "Session ID out"=w878:T4)  [unwired: 5 in]
                n226 = call <vilib>:"Call.vi"("Function or Method Name"="HPLC", "error in (no error)"=w874, "Python Object References In"=w876, "Session ID"=w878) -> ("error out"=w892:errorcluster, "Python Object References Out"=w883:T5, "Session ID out"=w884:T4)  [unwired: 5 in]
                n227 = call-poly <vilib>:"Unpack.vi"("error in (no error)"=w892, "Python Object References In"=w883, "Session ID"=w884) -> ("error out"=w893:errorcluster, "Value"=→"C BAcid 9":dbl, "Python Object References Out"=w888:T5, "Session ID out"=w887:T4)  [unwired: 5 in]
                n228 = call-poly <vilib>:"Unpack.vi"("error in (no error)"=w893, "Python Object References In"=w888, "Session ID"=w887) -> ("error out"=w894:errorcluster, "Value"=→"C EB 9":dbl, "Session ID out"=w889:T4)  [unwired: 5 in, 1 out]
                n229 = call <vilib>:"Close Session.vi"("error in (no error)"=w894, "Session ID"=w889) -> ()  [unwired: 9 in, 1 out]
              }
              frame #1 {
                # "Number read"
                n230 = call <vilib>:"New Session.vi"("Path to Python Module (.py File)"=path "C:/Users/User/Documents/LabVIEW Data/2015 Projects/Combined/closed_loop_benzoic_acid.py") -> ("error out"=w949:errorcluster, "Session ID out"=w948:T4)  [unwired: 9 in]
                n231 = call <vilib>:"Pack.vi"("Argument"=w944, "error in (no error)"=w949, "Session ID"=w948) -> ("error out"=w926:errorcluster, "Python Object References Out"=w928:T5, "Session ID out"=w930:T4)  [unwired: 6 in]
                n232 = call <vilib>:"Pack.vi"("Argument"=w924, "error in (no error)"=w926, "Python Object References In"=w928, "Session ID"=w930) -> ("error out"=w925:errorcluster, "Python Object References Out"=w927:T5, "Session ID out"=w929:T4)  [unwired: 5 in]
                n233 = call <vilib>:"Pack.vi"("Argument"=w923, "error in (no error)"=w925, "Python Object References In"=w927, "Session ID"=w929) -> ("error out"=w896:errorcluster, "Python Object References Out"=w899:T5, "Session ID out"=w901:T4)  [unwired: 5 in]
                n234 = call <vilib>:"Pack.vi"("Argument"=w895, "error in (no error)"=w896, "Python Object References In"=w899, "Session ID"=w901) -> ("error out"=w897:errorcluster, "Python Object References Out"=w898:T5, "Session ID out"=w900:T4)  [unwired: 5 in]
                n235 = call <vilib>:"Call.vi"("Function or Method Name"="design_next_experiment", "error in (no error)"=w897, "Python Object References In"=w898, "Session ID"=w900) -> ("error out"=w910:errorcluster, "Python Object References Out"=w913:T5, "Session ID out"=w916:T4)  [unwired: 5 in]
                n236 = call-poly <vilib>:"Unpack.vi"("error in (no error)"=w910, "Python Object References In"=w913, "Session ID"=w916) -> ("error out"=w909:errorcluster, "Value"=→"Temp 10":dbl, "Python Object References Out"=w912:T5, "Session ID out"=w915:T4)  [unwired: 5 in]
                n237 = call-poly <vilib>:"Unpack.vi"("error in (no error)"=w909, "Python Object References In"=w912, "Session ID"=w915) -> ("error out"=w908:errorcluster, "Value"=→"Flow 10":dbl, "Python Object References Out"=w911:T5, "Session ID out"=w914:T4)  [unwired: 5 in]
                n238 = call-poly <vilib>:"Unpack.vi"("error in (no error)"=w908, "Python Object References In"=w911, "Session ID"=w914) -> ("error out"=w902:errorcluster, "Value"=→"Conc 10":dbl, "Python Object References Out"=w903:T5, "Session ID out"=w904:T4)  [unwired: 5 in]
                n239 = call-poly <vilib>:"Unpack.vi"("error in (no error)"=w902, "Python Object References In"=w903, "Session ID"=w904) -> ("error out"=w954:errorcluster, "Value"=→"Param 1 9":dbl, "Python Object References Out"=w952:T5, "Session ID out"=w950:T4)  [unwired: 5 in]
                n240 = call-poly <vilib>:"Unpack.vi"("error in (no error)"=w954, "Python Object References In"=w952, "Session ID"=w950) -> ("error out"=w955:errorcluster, "Value"=→"T value 1 9":dbl, "Python Object References Out"=w953:T5, "Session ID out"=w951:T4)  [unwired: 5 in]
                n241 = call-poly <vilib>:"Unpack.vi"("error in (no error)"=w955, "Python Object References In"=w953, "Session ID"=w951) -> ("error out"=w956:errorcluster, "Value"=→"Param 2 9":dbl, "Python Object References Out"=w947:T5, "Session ID out"=w946:T4)  [unwired: 5 in]
                n242 = call-poly <vilib>:"Unpack.vi"("error in (no error)"=w956, "Python Object References In"=w947, "Session ID"=w946) -> ("error out"=w938:errorcluster, "Value"=→"T value 2 9":dbl, "Python Object References Out"=w940:T5, "Session ID out"=w942:T4)  [unwired: 5 in]
                n243 = call-poly <vilib>:"Unpack.vi"("error in (no error)"=w938, "Python Object References In"=w940, "Session ID"=w942) -> ("error out"=w937:errorcluster, "Value"=→"T Ref 9":dbl, "Python Object References Out"=w939:T5, "Session ID out"=w941:T4)  [unwired: 5 in]
                n244 = call-poly <vilib>:"Unpack.vi"("error in (no error)"=w937, "Python Object References In"=w939, "Session ID"=w941) -> ("error out"=w920:errorcluster, "Value"=→"Correlation 9":dbl, "Python Object References Out"=w921:T5, "Session ID out"=w922:T4)  [unwired: 5 in]
                n245 = call-poly <vilib>:"Unpack.vi"("error in (no error)"=w920, "Python Object References In"=w921, "Session ID"=w922) -> ("error out"=w934:errorcluster, "Value"=→"X2 9":dbl, "Python Object References Out"=w933:T5, "Session ID out"=w932:T4)  [unwired: 5 in]
                n246 = call-poly <vilib>:"Unpack.vi"("error in (no error)"=w934, "Python Object References In"=w933, "Session ID"=w932) -> ("error out"=w917:errorcluster, "Value"=→"X2 ref 9":dbl, "Session ID out"=w918:T4)  [unwired: 5 in, 1 out]
                n247 = call <vilib>:"Close Session.vi"("error in (no error)"=w917, "Session ID"=w918) -> ()  [unwired: 9 in, 1 out]
              }
            }
            "Exp Finish" <- TRUE
          }
        }
      }
      frame True {
        w961 = 0
      }
    }
    n248 = timed-loop {
      tunnel: w127 -> [w1115]
      tunnel: w126 -> [w1114]
      tunnel: [w1063] -> w125
      tunnel: [w1062] -> w124
      timing: w123 -> [_]
      timing-out: [_] -> w122
      tunnel: w121 -> [w1049]
      tunnel: w120 -> [w1053]
      tunnel: w119 -> [w1052]
      tunnel: [w1048] -> w118
      tunnel: [w1047] -> w117
      tunnel: [w1028] -> w116
      tunnel: w107 -> [w1044]
      tunnel: w106 -> [w966]
      tunnel: w105 -> [w985]
      tunnel: w115 -> [w1033]
      tunnel: w114 -> [w1032]
      tunnel: w113 -> [w1031]
      tunnel: w112 -> [w1030]
      shift-right: [w990] -> _
      shift-left: _ -> [w1022]
      tunnel: [w1025] -> w111
      tunnel: [w1024] -> w110
      tunnel: ["Stop everything"] -> w108
      tunnel: "Automated Experiments or Direct Control" -> [w991]
      tunnel: w94 -> [w980]
      tunnel: w93 -> [w979]
      tunnel: [w978] -> w92
      tunnel: [w977] -> w91
      i -> [w1013]
      stop <- w1020 stop-if-true
      w1029 = 9.0 ("Safety Shut Down Pressure (barg)")
      w1045 = 180
      # "in case out of range changes conc to within possible range"
      # "1st 4 flowrates\n5,6 temperatures\n7 pressure (1)\n8 gas (1)"
      # "temperature or syringe or pressure"
      # "We are graphing in barg"
      # "temperature or syringe"
      # "Empty Syringe has level of 50"
      n249 = node-c288() -> ()  [unwired: 1 in, 1 out]
      n250 = call-poly <vilib>:"DAQmx Read.vi"("task/channels in"=w980, "error in"=w979) -> ("task out"=w978:refnum<k21>, "data"=w973:dbl, "error out"=w977:errorcluster)  [unwired: 11 in]
      n251 = Multiply(x=5.1522, y=w973) -> (x*y=w976:dbl)
      n252 = Add(x=-2.6852, y=w976) -> (x+y=w969:dbl)
      "Liquid Inlet Pressure (bar g)" <- w969
      n253 = Greater?(x=w966, y=50) -> (0:w967:bool)
      n254 = Less?(x=w966, y=0) -> (x < y?=w964:bool)
      n255 = case shown="False" w967 {
        tunnel: [w1119 1] -> w963
        tunnel: w966 -> [w1119 _]
        frame False {
        }
        frame True {
        }
      }
      n256 = case shown="False" w964 {
        tunnel: [w1117 1] -> w962
        tunnel: w963 -> [w1117 _]
        frame False {
        }
        frame True {
        }
      }
      n257 = for {
        N: 4 -> [_]
        tunnel: w1115 -> [w1396] mode=indexing
        tunnel: [w1394] -> w1109 mode=indexing
        tunnel: [w1391] -> w1104 mode=indexing
        tunnel: [w1390] -> w1103 mode=indexing
        tunnel: [w1389] -> w1102 mode=indexing
        tunnel: w1114 -> [w1388] mode=indexing
        i -> [w1395]
        n258 = call "NCS_GetFlowRateIs.vi"("error in (no error)"=w1388, "dosingunit"=w1395, "device handle in"=w1396) -> ("error out"=w1392:errorcluster, "flowrate is"=w1394:dbl, "device handle out"=w1393:u32)
        n259 = call "NCS_GetSyringeLevelIs.vi"("error in (no error)"=w1392, "dosingunit"=w1395, "device handle in"=w1393) -> ("error out"=w1389:errorcluster, "syringe level is"=w1391:dbl, "device handle out"=w1390:u32)
      }
      n260 = Index Array(array=w1104, index=0) -> (element=w1017:dbl)
      "Syringe Level 1" <- w1017
      n261 = Index Array(array=w1104, index=3) -> (element=w1014:dbl)
      "Syringe Level 4" <- w1014
      n262 = Index Array(array=w1104, index=1) -> (element=w1016:dbl)
      "Syringe Level 2" <- w1016
      n263 = Index Array(array=w1104, index=2) -> (element=w1015:dbl)
      "Syringe Level 3" <- w1015
      n264 = case shown="True" "Shut down in empty?\nLeft off, right on" {
        tunnel: [FALSE w1290] -> w1018
        tunnel: w1017 -> [_ w1289]
        tunnel: w1016 -> [_ w1288]
        tunnel: w1015 -> [_ w1287]
        tunnel: w1014 -> [_ w1286]
        frame False {
        }
        frame True {
          w1291 = 50
          n265 = Less Or Equal?(x=w1288, y=w1291) -> (x <= y?=w1297:bool)
          n266 = Less Or Equal?(x=w1289, y=w1291) -> (x <= y?=w1292:bool)
          n267 = Less Or Equal?(x=w1287, y=w1291) -> (x <= y?=w1295:bool)
          n268 = Less Or Equal?(x=w1286, y=w1291) -> (x <= y?=w1293:bool)
          n269 = Or(x=w1292, y=w1297) -> (x .or. y?=w1296:bool)
          n270 = Or(x=w1296, y=w1295) -> (x .or. y?=w1294:bool)
          n271 = Or(x=w1294, y=w1293) -> (x .or. y?=w1290:bool)
        }
      }
      n272 = Index Array(array=w1109, index=0) -> (element=w1001:dbl)
      "Flowrate 1 Low" <- w1001
      n273 = Index Array(array=w1109, index=3) -> (element=w1003:dbl)
      "Flowrate 4 Ethanol" <- w1003
      n274 = Index Array(array=w1109, index=1) -> (element=w1000:dbl)
      "Flowrate 2 High" <- w1000
      n275 = Index Array(array=w1109, index=2) -> (element=w1004:dbl)
      "Flowrate 3 Acid" <- w1004
      n276 = case shown="True" "Clear" {
        tunnel: w1022 -> [w1298 _]
        tunnel: [w1298 w1299] -> w1021
        frame False {
        }
        frame True {
          n277 = Initialize Array(0, 1) -> (w1299:i32[])
        }
      }
      n278 = call-poly <vilib>:"DAQmx Read.vi"("task/channels in"=w1033, "error in"=w1032) -> ("task out"=w1025:refnum<k21>, "data"=w1038:dbl[], "error out"=w1024:errorcluster)  [unwired: 11 in]
      n279 = Add(x=w1001, y=w1000) -> (x+y=w1006:dbl)
      n280 = Add(x=w1006, y=w1004) -> (x+y=w1005:dbl)
      n281 = Index Array(array=w1038, index=0) -> (element=w1036:dbl)
      n282 = Add(x=w1005, y=w1003) -> (x+y=w1002:dbl)
      "Total Flowrate (uL/min)" <- w1002
      n283 = Divide(x=w1001, y=w1002) -> (x/y=w995:dbl)
      n284 = Multiply(x=w1036, y=w1031) -> (x*y=w1037:dbl)
      n285 = Multiply(x="Low Conc", y=w995) -> (x*y=w999:dbl)
      n286 = Add(x=w1037, y=w1030) -> (x+y=w1034:dbl)
      n287 = Divide(x=w1000, y=w1002) -> (x/y=w996:dbl)
      n288 = Multiply(x="High Conc", y=0.9) -> (x*y=w987:dbl)
      n289 = Multiply(x="Low Conc", y=0.9) -> (x*y=w986:dbl)
      n290 = Multiply(x="High Conc", y=w996) -> (x*y=w998:dbl)
      n291 = Add(x=w999, y=w998) -> (x+y=→"Feed Concentration (M)":dbl)
      n292 = In Range and Coerce(upper limit=w987, x=w985, lower limit=w986) -> (coerced(x)=w982:dbl, In Range?=w984:bool)
      n293 = case shown="True" w984 {
        tunnel: [w1122 w1124] -> w983
        tunnel: w985 -> [_ w1124]
        tunnel: w982 -> [w1122 _]
        tunnel: [TRUE FALSE] -> w981
        frame False {
        }
        frame True {
        }
      }
      "Desired Conc Not Possible" <- w981
      n294 = Multiply(x=w1034, y=0.0689476) -> (x*y=w970:dbl)
      "Gas Back Pressure (barg)" <- w970
      n295 = case shown="False" w991 {
        tunnel: [w1368 w1369] -> w1100
        tunnel: w962 -> [w1355 _]
        tunnel: w983 -> [w1357 _]
        tunnel: "High Conc" -> [w1354 _]
        tunnel: "Low Conc" -> [w1353 _]
        frame False {
          w1352 = 0.1
          # "swapped it so syringe 2 is high and 1 is low"
          n296 = Subtract(x=w1354, y=w1353) -> (x-y=w1364:dbl)
          n297 = Subtract(x=1, y=w1352) -> (x-y=w1360:dbl)
          n298 = Divide(x=w1357, y=w1360) -> (x/y=w1366:dbl)
          n299 = Multiply(x=0, y=w1355) -> (x*y=w1350:dbl)
          n300 = Subtract(x=w1354, y=w1366) -> (x-y=w1363:dbl)
          n301 = Subtract(x=w1366, y=w1353) -> (x-y=w1365:dbl)
          n302 = Divide(x=w1365, y=w1364) -> (x/y=w1362:dbl)
          n303 = Divide(x=w1363, y=w1364) -> (x/y=w1361:dbl)
          n304 = Multiply(x=w1362, y=w1360) -> (x*y=w1359:dbl)
          n305 = Multiply(x=w1361, y=w1360) -> (x*y=w1358:dbl)
          n306 = Multiply(x=w1355, y=w1358) -> (x*y=w1348:dbl)
          n307 = Multiply(x=w1355, y=w1359) -> (x*y=w1349:dbl)
          n308 = Multiply(x=w1355, y=w1352) -> (x*y=w1351:dbl)
          n309 = Build Array(w1348, w1349, w1351, w1350) -> (w1368:dbl[])
          "Volumetric Fraction Acid" <- w1352
        }
        frame True {
          n310 = Build Array("Set Flowrate 1", "Set Flowrate 2", "Set Flowrate 3", "Set Flowrate 4") -> (w1369:dbl[])
        }
      }
      n311 = Build Array (concatenate)(w1021, w970) -> (w990:dbl[])
      "Calculated Pressure" <- w990
      n312 = Greater Or Equal?(x=w970, y=w1029) -> (x >= y?=w1026:bool)
      n313 = case shown="True" w991 {
        tunnel: [w1303 FALSE] -> w993
        tunnel: w1013 -> [w1302 _]
        frame False {
          # "changes set points for each new exp"
          n314 = Equal?(x=w1302, y=0) -> (x = y?=w1303:bool)
        }
        frame True {
          # "at end of each exp"
          # "doesnt automatically change set point"
        }
      }
      n315 = Or(x=w993, y="Update Temperature Set Point") -> (x .or. y?=w1055:bool)
      n316 = case shown="True" w1055 {
        tunnel: w1053 -> [w1307 w1315]
        tunnel: w1052 -> [w1306 w1314]
        tunnel: [w1307 w1313] -> w1051
        tunnel: [w1306 w1312] -> w1050
        tunnel: w1049 -> [_ w1311]
        tunnel: w991 -> [_ w1309]
        tunnel: w1044 -> [_ w1308]
        frame False {
        }
        frame True {
          n317 = case shown="True" w1309 {
            tunnel: [w1316 "Set Point (oC)"] -> w1310
            tunnel: w1308 -> [w1316 _]
            frame False {
            }
            frame True {
            }
          }
          n318 = call "CN7500_Write Set Point Value.vi"("Target Set Point Value"=w1310, "error in (no error)"=w1314, "Controller Number"=w1311, "VISA In"=w1315) -> ("error out"=w1312:errorcluster, "VISA Out"=w1313:refnum<visa-resource-name>)  [unwired: 6 in]
        }
      }
      n319 = Or(x="Generate Flow", y=w993) -> (x .or. y?=w994:bool)
      n320 = case shown="True" w994 {
        tunnel: w1103 -> [w1375 w1380]
        tunnel: w1102 -> [w1374 w1379]
        tunnel: [w1374 w1378] -> w1008
        tunnel: [w1375 w1377] -> w1007
        tunnel: w1100 -> [_ w1376]
        frame False {
        }
        frame True {
          n321 = for {
            N: 4 -> [_]
            tunnel: w1380 -> [w1387] mode=indexing
            tunnel: w1379 -> [w1386] mode=indexing
            tunnel: [w1385] -> w1378 mode=indexing
            tunnel: [w1384] -> w1377 mode=indexing
            tunnel: w1376 -> [w1382] mode=indexing
            i -> [w1383]
            n322 = call "NCS_GenerateFlow.vi"("error in (no error)"=w1386, "flowrate"=w1382, "dosingunit"=w1383, "device handle in"=w1387) -> ("error out"=w1385:errorcluster, "device handle out"=w1384:u32)
          }
        }
      }
      n323 = call "CN7500_Read Process Value.vi"("error in (no error)"=w1050, "Controller Number"=w1049, "VISA In"=w1051) -> ("error out"=w1048:errorcluster, "Set Point Value"=w1040:dbl, "Process Value"=w1041:dbl, "VISA Out"=w1047:refnum<visa-resource-name>)  [unwired: 5 in]
      "Temp Set Point (oC)" <- w1040
      "Actual Temp (oC)" <- w1041
      n324 = Merge Signals(w1041, w1040) -> (→"Temperature":dynamicdata)
      n325 = Merge Signals(w1001, w1000, w1004, w1003, w1041, w1040, w970, w969) -> (w1061:dynamicdata)
      n326 = Greater Or Equal?(x=w1041, y=w1045) -> (x >= y?=w1043:bool)
      n327 = call "Write To Measurement File"("Signals"=w1061) -> ()  [unwired: 16 in, 3 out]
      n328 = Index Array(array=w1008, index=0) -> (element=w1090:errorcluster)
      n329 = Index Array(array=w1007, index=0) -> (element=w1091:u32)
      n330 = Index Array(array=w1008, index=3) -> (element=w1080:errorcluster)
      n331 = Index Array(array=w1008, index=2) -> (element=w1082:errorcluster)
      n332 = Index Array(array=w1008, index=1) -> (element=w1084:errorcluster)
      n333 = Index Array(array=w1007, index=3) -> (element=w1081:u32)
      n334 = Index Array(array=w1007, index=2) -> (element=w1083:u32)
      n335 = Index Array(array=w1007, index=1) -> (element=w1085:u32)
      n336 = case shown="False" "Stop Dose 2" {
        tunnel: w1085 -> [w1335 w1340]
        tunnel: w1084 -> [w1334 w1339]
        tunnel: [w1335 w1338] -> w1077
        tunnel: [w1334 w1337] -> w1076
        frame False {
        }
        frame True {
          n337 = call "NCS_Stop.vi"("error in (no error)"=w1339, "dosingunit"=1, "device handle in"=w1340) -> ("error out"=w1337:errorcluster, "device handle out"=w1338:u32)
        }
      }
      n338 = case shown="False" "Stop Dose 1" {
        tunnel: w1091 -> [w1342 w1347]
        tunnel: w1090 -> [w1341 w1346]
        tunnel: [w1342 w1345] -> w1079
        tunnel: [w1341 w1344] -> w1078
        frame False {
        }
        frame True {
          n339 = call "NCS_Stop.vi"("error in (no error)"=w1346, "dosingunit"=0, "device handle in"=w1347) -> ("error out"=w1344:errorcluster, "device handle out"=w1345:u32)
        }
      }
      n340 = case shown="False" "Stop Dose 3" {
        tunnel: w1083 -> [w1328 w1333]
        tunnel: w1082 -> [w1327 w1332]
        tunnel: [w1328 w1331] -> w1075
        tunnel: [w1327 w1330] -> w1074
        frame False {
        }
        frame True {
          n341 = call "NCS_Stop.vi"("error in (no error)"=w1332, "dosingunit"=2, "device handle in"=w1333) -> ("error out"=w1330:errorcluster, "device handle out"=w1331:u32)
        }
      }
      n342 = case shown="False" "Stop Dose 4" {
        tunnel: w1081 -> [w1321 w1326]
        tunnel: w1080 -> [w1320 w1325]
        tunnel: [w1321 w1324] -> w1073
        tunnel: [w1320 w1323] -> w1072
        frame False {
        }
        frame True {
          n343 = call "NCS_Stop.vi"("error in (no error)"=w1325, "dosingunit"=3, "device handle in"=w1326) -> ("error out"=w1323:errorcluster, "device handle out"=w1324:u32)
        }
      }
      n344 = case shown="False" "Safety or Emergency Syringe Control" {
        tunnel: w1079 -> [w1132 w1173]
        tunnel: w1078 -> [w1128 w1172]
        tunnel: w1077 -> [w1131 w1171]
        tunnel: w1076 -> [w1127 w1170]
        tunnel: w1075 -> [w1130 w1169]
        tunnel: w1074 -> [w1126 w1168]
        tunnel: w1073 -> [w1129 w1167]
        tunnel: w1072 -> [w1125 w1166]
        tunnel: [w1132 w1143] -> w1071
        tunnel: [w1131 w1142] -> w1070
        tunnel: [w1130 w1141] -> w1069
        tunnel: [w1129 w1140] -> w1068
        tunnel: [w1127 w1139] -> w1067
        tunnel: [w1126 w1138] -> w1066
        tunnel: [w1125 w1137] -> w1065
        tunnel: [w1128 w1133] -> w1064
        frame False {
        }
        frame True {
          n345 = case shown="False" "Calibrate 2" {
            tunnel: w1171 -> [w1272 w1277]
            tunnel: w1170 -> [w1271 w1276]
            tunnel: [w1272 w1275] -> w1160
            tunnel: [w1271 w1274] -> w1159
            frame False {
            }
            frame True {
              n346 = call "NCS_Calibrate.vi"("error in (no error)"=w1276, "dosingunit"=1, "device handle in"=w1277) -> ("error out"=w1274:errorcluster, "device handle out"=w1275:u32)
            }
          }
          n347 = case shown="False" "Calibrate 3" {
            tunnel: w1169 -> [w1265 w1270]
            tunnel: w1168 -> [w1264 w1269]
            tunnel: [w1265 w1268] -> w1158
            tunnel: [w1264 w1267] -> w1157
            frame False {
            }
            frame True {
              n348 = call "NCS_Calibrate.vi"("error in (no error)"=w1269, "dosingunit"=2, "device handle in"=w1270) -> ("error out"=w1267:errorcluster, "device handle out"=w1268:u32)
            }
          }
          n349 = case shown="False" "Calibrate 1" {
            tunnel: w1173 -> [w1279 w1284]
            tunnel: w1172 -> [w1278 w1283]
            tunnel: [w1279 w1282] -> w1162
            tunnel: [w1278 w1281] -> w1161
            frame False {
            }
            frame True {
              n350 = call "NCS_Calibrate.vi"("error in (no error)"=w1283, "dosingunit"=0, "device handle in"=w1284) -> ("error out"=w1281:errorcluster, "device handle out"=w1282:u32)
            }
          }
          n351 = case shown="False" "Calibrate 4" {
            tunnel: w1167 -> [w1258 w1263]
            tunnel: w1166 -> [w1257 w1262]
            tunnel: [w1258 w1261] -> w1156
            tunnel: [w1257 w1260] -> w1155
            frame False {
            }
            frame True {
              n352 = call "NCS_Calibrate.vi"("error in (no error)"=w1262, "dosingunit"=3, "device handle in"=w1263) -> ("error out"=w1260:errorcluster, "device handle out"=w1261:u32)
            }
          }
          n353 = case shown="False" "Empty 2" {
            tunnel: w1160 -> [w1238 w1242]
            tunnel: w1159 -> [w1237 w1240]
            tunnel: [w1238 w1241] -> w1146
            tunnel: [w1237 w1239] -> w1147
            frame False {
            }
            frame True {
              w1244 = 1
              n354 = call "NCS_GetFlowRateMax.vi"("error in (no error)"=w1240, "dosingunit"=w1244, "device handle in"=w1242) -> ("error out"=w1245:errorcluster, "flow rate max"=w1243:dbl, "device handle out"=w1246:u32)
              n355 = call "NCS_EmptySyrige.vi"("error in (no error)"=w1245, "flowrate"=w1243, "dosingunit"=w1244, "device handle in"=w1246) -> ("error out"=w1239:errorcluster, "device handle out"=w1241:u32)
            }
          }
          n356 = case shown="False" "Empty 1" {
            tunnel: w1162 -> [w1248 w1256]
            tunnel: w1161 -> [w1247 w1253]
            tunnel: [w1248 w1254] -> w1144
            tunnel: [w1247 w1251] -> w1145
            frame False {
            }
            frame True {
              w1250 = 0
              n357 = call "NCS_GetFlowRateMax.vi"("error in (no error)"=w1253, "dosingunit"=w1250, "device handle in"=w1256) -> ("error out"=w1252:errorcluster, "flow rate max"=w1249:dbl, "device handle out"=w1255:u32)
              n358 = call "NCS_EmptySyrige.vi"("error in (no error)"=w1252, "flowrate"=w1249, "dosingunit"=w1250, "device handle in"=w1255) -> ("error out"=w1251:errorcluster, "device handle out"=w1254:u32)
            }
          }
          n359 = case shown="False" "Empty 3" {
            tunnel: w1158 -> [w1228 w1229]
            tunnel: w1157 -> [w1227 w1230]
            tunnel: [w1228 w1231] -> w1148
            tunnel: [w1227 w1232] -> w1149
            frame False {
            }
            frame True {
              w1234 = 2
              n360 = call "NCS_GetFlowRateMax.vi"("error in (no error)"=w1230, "dosingunit"=w1234, "device handle in"=w1229) -> ("error out"=w1235:errorcluster, "flow rate max"=w1233:dbl, "device handle out"=w1236:u32)
              n361 = call "NCS_EmptySyrige.vi"("error in (no error)"=w1235, "flowrate"=w1233, "dosingunit"=w1234, "device handle in"=w1236) -> ("error out"=w1232:errorcluster, "device handle out"=w1231:u32)
            }
          }
          n362 = case shown="False" "Empty 4" {
            tunnel: w1156 -> [w1218 w1219]
            tunnel: w1155 -> [w1217 w1220]
            tunnel: [w1218 w1222] -> w1150
            tunnel: [w1217 w1221] -> w1151
            frame False {
            }
            frame True {
              w1224 = 3
              n363 = call "NCS_GetFlowRateMax.vi"("error in (no error)"=w1220, "dosingunit"=w1224, "device handle in"=w1219) -> ("error out"=w1225:errorcluster, "flow rate max"=w1223:dbl, "device handle out"=w1226:u32)
              n364 = call "NCS_EmptySyrige.vi"("error in (no error)"=w1225, "flowrate"=w1223, "dosingunit"=w1224, "device handle in"=w1226) -> ("error out"=w1221:errorcluster, "device handle out"=w1222:u32)
            }
          }
          n365 = case shown="False" "Refill 2" {
            tunnel: w1146 -> [w1198 w1202]
            tunnel: w1147 -> [w1197 w1200]
            tunnel: [w1198 w1201] -> w1142
            tunnel: [w1197 w1199] -> w1139
            frame False {
            }
            frame True {
              w1204 = 1
              n366 = call "NCS_GetFlowRateMax.vi"("error in (no error)"=w1200, "dosingunit"=w1204, "device handle in"=w1202) -> ("error out"=w1205:errorcluster, "flow rate max"=w1203:dbl, "device handle out"=w1206:u32)
              n367 = call "NCS_RefillSyrige.vi"("error in (no error)"=w1205, "flowrate"=w1203, "dosingunit"=w1204, "device handle in"=w1206) -> ("error out"=w1199:errorcluster, "device handle out"=w1201:u32)
            }
          }
          n368 = case shown="False" "Refill 1" {
            tunnel: w1144 -> [w1208 w1216]
            tunnel: w1145 -> [w1207 w1213]
            tunnel: [w1208 w1214] -> w1143
            tunnel: [w1207 w1211] -> w1133
            frame False {
            }
            frame True {
              w1210 = 0
              n369 = call "NCS_GetFlowRateMax.vi"("error in (no error)"=w1213, "dosingunit"=w1210, "device handle in"=w1216) -> ("error out"=w1212:errorcluster, "flow rate max"=w1209:dbl, "device handle out"=w1215:u32)
              n370 = call "NCS_RefillSyrige.vi"("error in (no error)"=w1212, "flowrate"=w1209, "dosingunit"=w1210, "device handle in"=w1215) -> ("error out"=w1211:errorcluster, "device handle out"=w1214:u32)
            }
          }
          n371 = case shown="False" "Refill 3" {
            tunnel: w1148 -> [w1188 w1189]
            tunnel: w1149 -> [w1187 w1190]
            tunnel: [w1188 w1191] -> w1141
            tunnel: [w1187 w1192] -> w1138
            frame False {
            }
            frame True {
              w1194 = 2
              n372 = call "NCS_GetFlowRateMax.vi"("error in (no error)"=w1190, "dosingunit"=w1194, "device handle in"=w1189) -> ("error out"=w1195:errorcluster, "flow rate max"=w1193:dbl, "device handle out"=w1196:u32)
              n373 = call "NCS_RefillSyrige.vi"("error in (no error)"=w1195, "flowrate"=w1193, "dosingunit"=w1194, "device handle in"=w1196) -> ("error out"=w1192:errorcluster, "device handle out"=w1191:u32)
            }
          }
          n374 = case shown="False" "Refill 4" {
            tunnel: w1150 -> [w1178 w1179]
            tunnel: w1151 -> [w1177 w1180]
            tunnel: [w1178 w1182] -> w1140
            tunnel: [w1177 w1181] -> w1137
            frame False {
            }
            frame True {
              w1184 = 3
              n375 = call "NCS_GetFlowRateMax.vi"("error in (no error)"=w1180, "dosingunit"=w1184, "device handle in"=w1179) -> ("error out"=w1185:errorcluster, "flow rate max"=w1183:dbl, "device handle out"=w1186:u32)
              n376 = call "NCS_RefillSyrige.vi"("error in (no error)"=w1185, "flowrate"=w1183, "dosingunit"=w1184, "device handle in"=w1186) -> ("error out"=w1181:errorcluster, "device handle out"=w1182:u32)
            }
          }
        }
      }
      n377 = Or(x=w1043, y=w1018) -> (x .or. y?=w1027:bool)
      n378 = Or(x=w1027, y=w1026) -> (x .or. y?=w1028:bool)
      n379 = Multiply(x="Minutes between Exp", y=60) -> (x*y=w1010:dbl)
      n380 = Divide(x=w1010, y=5) -> (x/y=w1011:dbl)
      n381 = Greater Or Equal?(x=w1013, y=w1011) -> (x >= y?=w1057:bool)
      n382 = Or(x=w1057, y=w1028) -> (x .or. y?=w1042:bool)
      n383 = Or(x="Skip Exp", y=w1042) -> (x .or. y?=w1058:bool)
      n384 = Or(x="Stop everything", y=w1058) -> (x .or. y?=w1020:bool)
      n385 = node-c288() -> ()  [unwired: 1 in, 1 out]
      n386 = Build Array(w1071, w1070, w1069, w1068) -> (w1063:u32[])
      n387 = Build Array(w1064, w1067, w1066, w1065) -> (w1062:errorcluster[])
      "loop ind" <- w1013
      "Safety Shut Down Temp" <- w1045
      "Safety Shut Down Pressure (barg)" <- w1029
    }
    n388 = Or(x=w108, y=w116) -> (x .or. y?=w109:bool)
    n389 = node-c288(w122) -> ()  [unwired: 1 out]
  }
  n390 = call <vilib>:"DAQmx Stop Task.vi"("task/channels in"=w16, "error in"=w15) -> ("task out"=w18:refnum<k21>, "error out"=w17:errorcluster)  [unwired: 12 in]
  n391 = Index Array(array=w45, index=0) -> (element=w47:u32)
  n392 = Index Array(array=w44, index=0) -> (element=w46:errorcluster)
  n393 = call <vilib>:"DAQmx Stop Task.vi"("task/channels in"=w5, "error in"=w3) -> ("task out"=w4:refnum<k21>, "error out"=w6:errorcluster)  [unwired: 12 in]
  n394 = call <vilib>:"DAQmx Clear Task.vi"("task in"=w18, "error in"=w17) -> ()  [unwired: 13 in, 1 out]
  n395 = call <vilib>:"DAQmx Clear Task.vi"("task in"=w4, "error in"=w6) -> ()  [unwired: 13 in, 1 out]
  n396 = call "NCS_CloseDevice.vi"("error in (no error)"=w46, "device handle"=w47) -> ()  [unwired: 1 out]
  n397 = call "CN7500_Write Set Point Value.vi"("Target Set Point Value"=25, "error in (no error)"=w33, "Controller Number"=w36, "VISA In"=w32) -> ("error out"=w38:errorcluster, "VISA Out"=w39:refnum<visa-resource-name>)  [unwired: 6 in]
  n398 = call "CN7500_Close.vi"("error in (no error)"=w38, "VISA resource name"=w39) -> ()  [unwired: 9 in, 1 out]
